vi "Q14070-Z060Abak.vi"() -> ()   [LabVIEW 2013]
uses:
  <vilib>/Utility/error.llb/whitespace.ctl
  <vilib>/Utility/file.llb/Read From Spreadsheet File (string).vi
  <vilib>/express/express arith-compare/Formula/XNode/ExpressFormulaBlockNode.xnode
  PCI8622_32.dll
  <vilib>/printing/EasyPrintingControls.llb/contents.ctl
  <vilib>/Utility/NIReport.llb/NI_ReportGenerationCore.lvlib
  <vilib>/printing/EasyPrintingControls.llb/report_type.ctl
  <vilib>/printing/EasyPrinting.llb/Easy Print VI Panel or Documentation (path).vi
  <vilib>/Utility/NIReport.llb/NI_report.lvclass
panel:
  in  "机械间隙值":dbl=3.5
  out "最大轴向力标准(N)":dbl=200.0 caption="L+Lmax(mm)" format="%#.3f"
  out "右平均轴向力(N)":dbl caption="L+Lmax(mm)" format="%#.3f"
  out "左平均轴向力(N)":dbl caption="最大位移偏离Lmax(mm)" format="%#.3f"
  out "员工ID":string
  out "急停":bool
  out "报警":dbl
  out "报警提示":string
  out "DeviceHandle":u32
  in  "设定轴向力调整次数":dbl=6.0
  out "出支线工步号":u32
  in  "最小间隙(mm)":dbl=0.001 format="%#.3f"
  in  "测头气缸右移":bool
  in  "测头气缸左移":bool
  in  "轴向力已做次数":dbl
  out "全行程间隙及轴向力合格":bool
  out "轴向力启动":bool
  out "间隙启动":bool
  in  "夹头松开":bool
  in  "夹头夹紧":bool
  out "找帽扭矩":dbl=8.0 caption="压力传感器" format="%#.2f"
  out "error out":errorcluster
  out "型号数量":i32
  out "error out 4":errorcluster
  in  "设定间隙调整次数":dbl=6.0
  out "读取产品ID":string
  out "下工位备料":bool
  out "下工位测试":bool
  out "下工位自动":bool
  out "下工位备料H":bool
  out "下工位测试H":bool
  out "下工位自动H":bool
  out "FGCS":string
  out "KSJJ":string
  out "Z060ARFID":string
  out "轴向力Y":dbl[](array[numeric])
  out "轴向力X":dbl[](array[numeric])
  out "间隙X数组":dbl[](array[numeric])
  out "间隙Y数组":dbl[](array[numeric])
  out "error out 3":errorcluster caption="错误输出"
  out "rfid工步号":u32
  out "芯片ID":string="201209190001"
  out "rfid完成":bool
  out "rfid触发":bool
  out "本序已做":bool
  in  "回零完成":bool
  in  "电动缸回零":bool
  in  "已调试次数":dbl
  in  "需调整角度(度)":dbl
  in  "转向器中心":dbl
  out "扭矩到达":bool
  out "黄灯":bool
  out "红灯":bool
  in  "基准位移":dbl caption="压力传感器" format="%#.3f"
  out "上序不合格":bool
  out "单点间隙合格":bool
  out "上序合格":bool
  out "测头机构电机":u32
  out "复位":bool
  in  "型号选择":u16(ring)=1 items=["J709", "J728", "J706"]
  in  "联线按钮":bool
  in  "工步号":u32
  in  "产品ID":string="201209190001"
  out "间隙位移(mm)":dbl caption="压力传感器" format="%#.3f"
  out "齿条推拉力(N)":dbl format="%#.2f"
  out "齿条扭矩(Nm)":dbl format="%#.2f"
  out "通讯状态":bool
  in  "员工ID":string
  out "员工姓名":string
  out "工步提示":string
  out "ADODB._Connection Out 2":refnum<k7>
  out "旋转齿条电机":u32
  out "电动缸电机":u32
  in  "停止":bool
  in  "参数加载":bool
  in  "选项卡控件":T1(tab)
  out "扭动曲线":cluster{"Y":dbl[], "Y":dbl[]}[](graph) caption="压球涨堵头1"
  out "中间位置间隙":dbl caption="间隙值L(mm)" format="%_2f"
  in  "中间间隙标准(mm)":dbl=0.07 format="%#.3f"
  in  "找帽OK":bool
  in  "全行程180°外间隙标准(mm)":dbl=0.1 format="%#.3f"
  out "右180°外全行程间隙":dbl caption="正向最大间隙L1(mm)" format="%_2f"
  out "左180°外全行程间隙":dbl caption="正向最大间隙L1(mm)" format="%_2f"
  out "右180°内全行程间隙":dbl caption="正向最大间隙L1(mm)" format="%_2f"
  out "左180°内全行程间隙":dbl caption="正向最大间隙L1(mm)" format="%_2f"
  in  "全行程180°内间隙标准(mm)":dbl=0.07 format="%_1f"
  out "左全行程间隙":dbl caption="正向最大间隙L1(mm)" format="%#.3f"
  out "右全行程间隙":dbl caption="正向最大间隙L1(mm)" format="%#.3f"
  out "总圈数最大值":dbl
  out "总圈数标准":dbl
  out "总行程最大值":dbl
  out "总行程标准(mm)":dbl
  out "平均轴向力MAX(N)":dbl=200.0 caption="L+Lmax(mm)" format="%#.3f"
  out "力波动标准(N)":dbl=60.0 caption="L+Lmax(mm)" format="%#.3f"
  out "轴向力标准(N)":dbl=100.0 caption="L+Lmax(mm)" format="%#.3f"
  out "右最大轴向力(N)":dbl caption="L+Lmax(mm)" format="%#_5f"
  out "左轴向力波动(N)":dbl caption="最大位移偏离Lmax(mm)" format="%#_4f"
  out "左最大轴向力(N)":dbl caption="最大位移偏离Lmax(mm)" format="%#_5f"
  out "行程跳动曲线":cluster{"Y":dbl[], "Y":dbl[]}[](graph) caption="压球涨堵头1"
  out "右轴向力波动(N)":dbl format="%#_4f"
  out "总行程(mm)":dbl format="%#_5f"
  out "总圈数":dbl format="%#.2f"
  in  "不合格品":bool
  in  "扭矩停止值":dbl=16.0
  in  "齿条右极限":dbl=-70.0 caption="压力传感器" format="%#.2f"
  in  "齿条左极限":dbl=-262.0 caption="压力传感器" format="%#.2f"
  in  "齿条移动速度":dbl=5.0 caption="压力传感器" format="%#.2f"
  in  "旋转伺服找帽转速":dbl=5.0 caption="压力传感器" format="%#.2f"
  in  "测量点扭矩":dbl=4.0 caption="压力传感器" format="%#.2f"
  in  "旋转伺服测量转速":dbl caption="压力传感器" format="%#.2f"
  in  "测头机构轴后退位":dbl=30.0 caption="压力传感器" format="%#.2f"
  in  "测头机构轴待检位":dbl caption="压力传感器" format="%#.2f"
  in  "测头机构轴检测位":dbl caption="压力传感器" format="%#.2f"
  in  "测头机构轴移动速度":dbl caption="压力传感器" format="%#.2f"
  out "点胶":bool
  in  "夹头松开":bool
  in  "夹头夹紧":bool
  in  "测头气缸右移":bool
  in  "测头气缸左移":bool
  in  "支线下降":bool
  in  "支线顶升":bool
  in  "出支线":bool
  in  "进支线":bool
  in  "主线下降":bool
  in  "主线顶升":bool
  in  "下阻挡器放行":bool
  in  "上阻挡器放行":bool
  out "夹头夹紧位":bool
  out "测头左位":bool
  out "测头右位":bool
  out "夹头松开":bool
  out "记号笔":bool
  in  "测头机构轴使能":bool
  in  "测头机构轴后退":bool
  in  "测头机构轴前进":bool
  in  "电动缸速度(mm/s)":dbl=10.0 format="%#.3f"
  out "电动缸位置(mm)":dbl=10000.0 format="%#.3f"
  in  "旋转伺服速度(°/s)":dbl=10.0 format="%#.3f"
  out "旋转伺服位置(°)":dbl=10000.0 format="%#.3f"
  in  "测头机构轴速度(mm/s)":dbl=10.0 format="%#.3f"
  out "测头机构轴位置(mm)":dbl=10000.0 format="%#.3f"
  in  "旋转齿条轴右转":bool
  in  "旋转齿条轴左转":bool
  in  "旋转齿条轴使能":bool
  in  "电动缸后退":bool
  in  "电动缸使能":bool
  in  "电动缸前进":bool
  in  "齿条扭矩比例偏移":dbl=1.0 format="%#.2f"
  in  "齿条扭矩零点偏移":dbl format="%#.2f"
  in  "齿条推拉力比例偏移":dbl=1.0 format="%#.2f"
  in  "齿条推拉力零点偏移":dbl format="%#.2f"
  in  "间隙位移比例偏移":dbl=1.0 format="%#.2f"
  in  "间隙位移零点偏移":dbl format="%#.2f"
  in  "传感器参数保存":bool
  in  "参数修改":bool
  in  "参数查询":bool
  in  "参数浏览表":string[][](table)
  # "芜湖机械转向器装配线"
  # "间隙及轴向力检测"
  # "Q14070机械转向器装配线"
  # "湖北唯思凌科装备制造有限公司 设计开发 (C)2015"
  # "≤"
  # "间隙测量判定值"
  # "间隙测量结果"
  # "≤"
  # "≤"
  # "≤"
  # "轴向力测量结果"
  # "轴向力测量标准"
  # "≤"
  # "≥"
  # "≤"
  # "≥"
  # "≤"
  # "≥"
  # "≤"
  # "不得大于20NM"
  # "传感器校验区"
  # "关于传感器校验：\n1、传感器校验需要由具备资质的单位或部门进行校验。\n2、具备权限的用户才能够修改传感器校验参数和试验参数。\n3、修改校验参数方法：先将比例偏移置为1，修改零点偏移，使零点值与校验的传感器一致；然后根据增幅调整比例偏移。"
  # "注意：\n具备权限的用户才能够修改传感器校验参数和试验参数！"
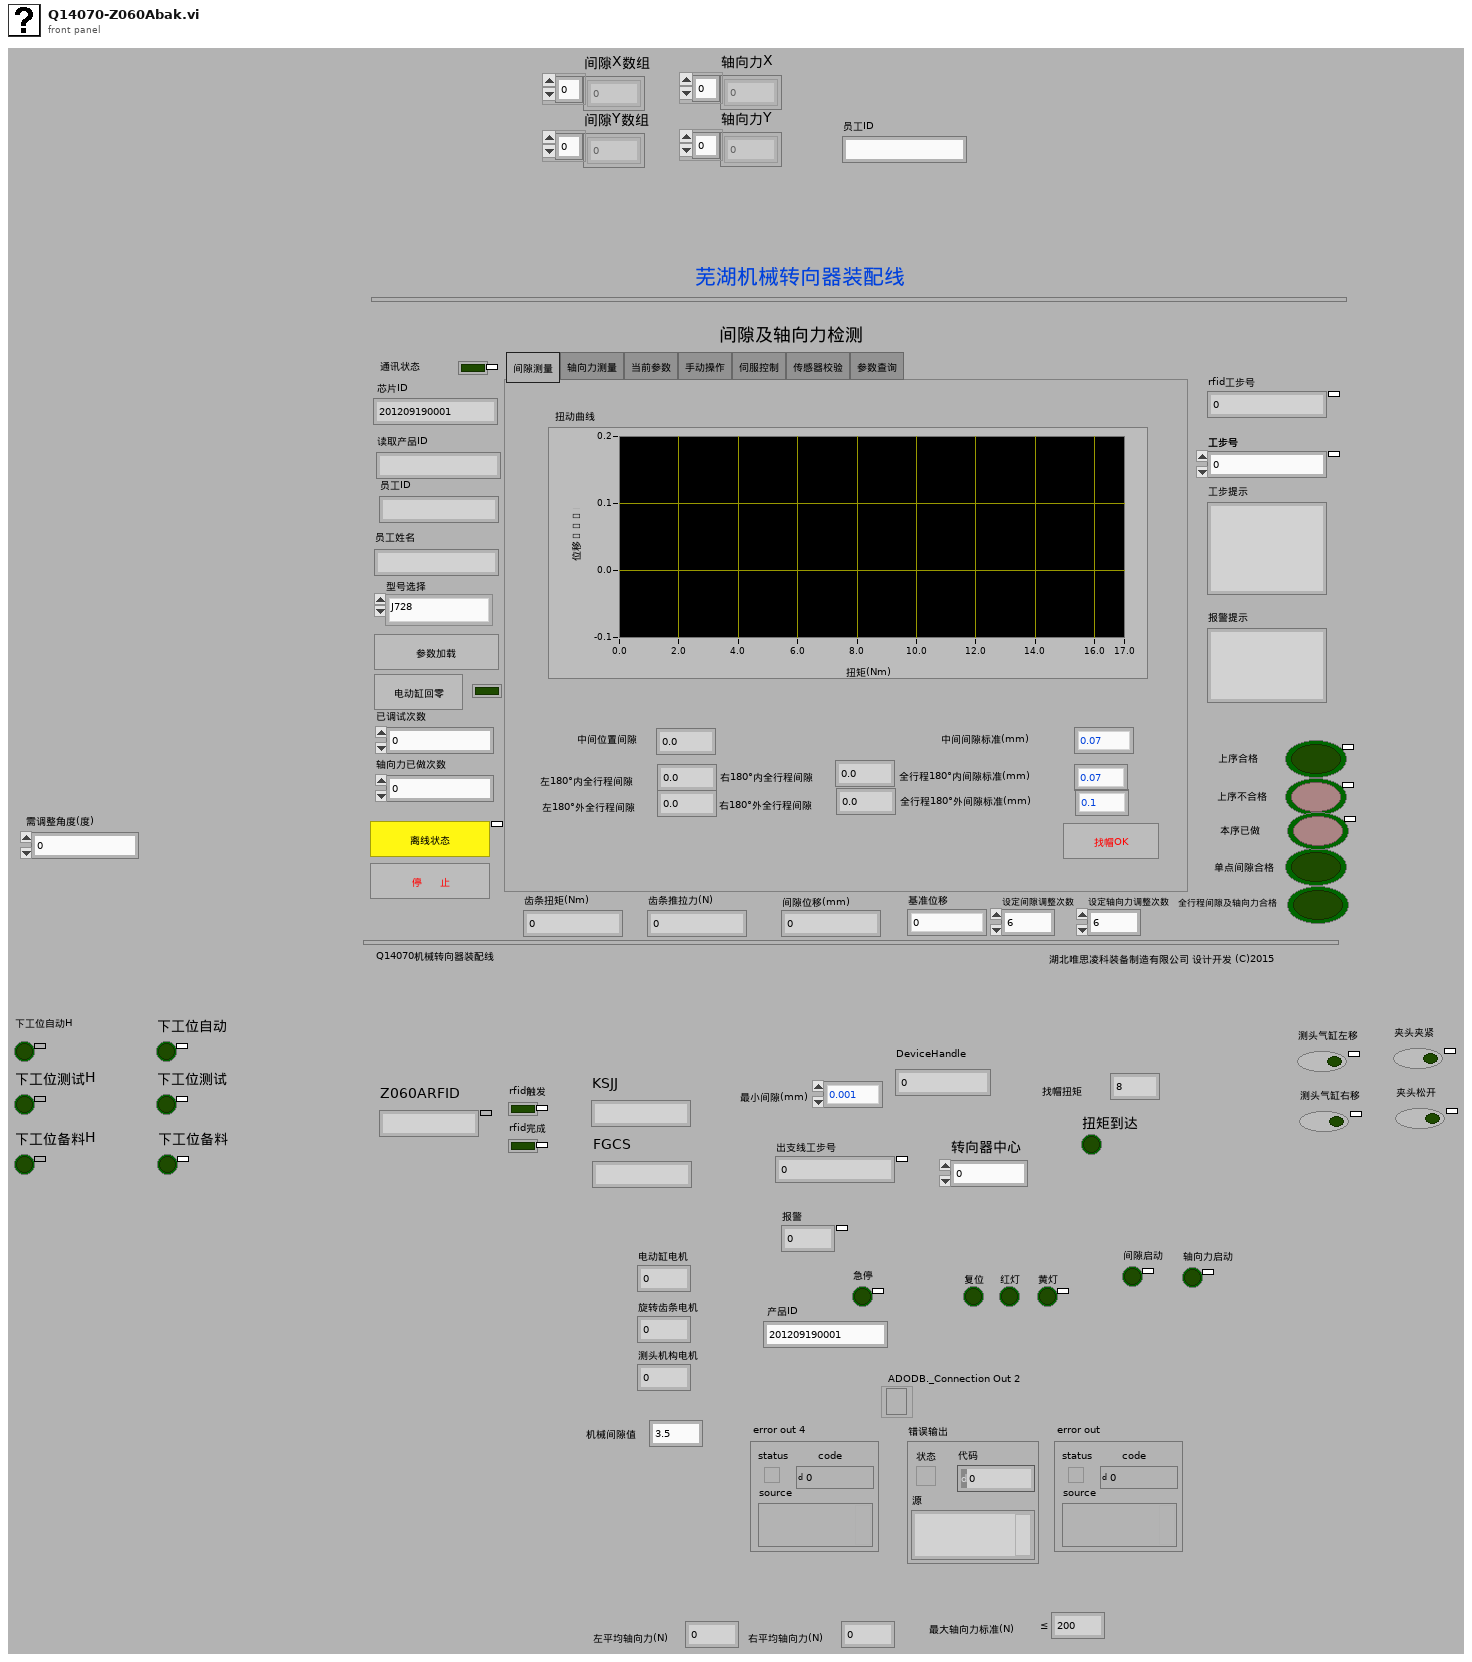
[diagram p1: front panel]
types:
  T1 = enum32{"间隙测量", "轴向力测量", "当前参数", "手动操作", "伺服控制", "传感器校验", "参数查询"}
  T2 = typedef "NI_ReportGenerationCore.lvlib/report_type.ctl" = u16
  T3 = typedef "NI_ReportGenerationCore.lvlib/contents.ctl" = u16
  T4 = typedef "imagedata.ctl" = cluster{"image type":i32, "image depth":i32, "image":u8[], "mask":u8[], "colors":u32[], "Rectangle":cluster{"left":i16, "top":i16, "right":i16, "bottom":i16}}
  T5 = enum8{"Enabled", "Disabled", "Disabled and Grayed Out"}
  T6 = typedef "whitespace.ctl" = u16
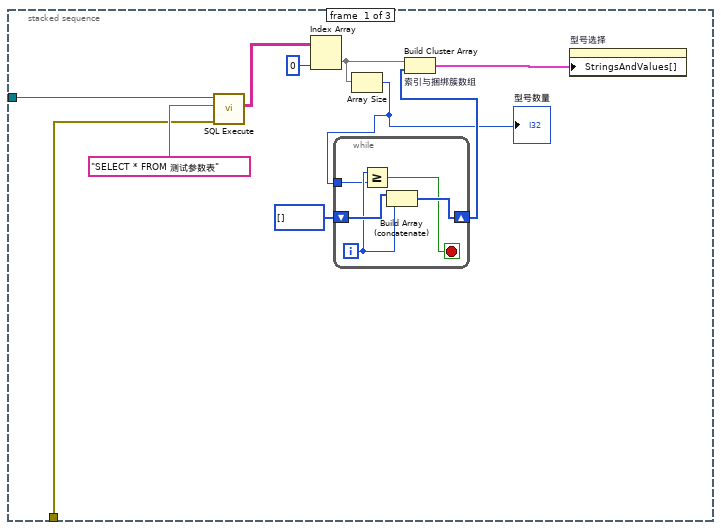
[diagram p4: hidden frame]
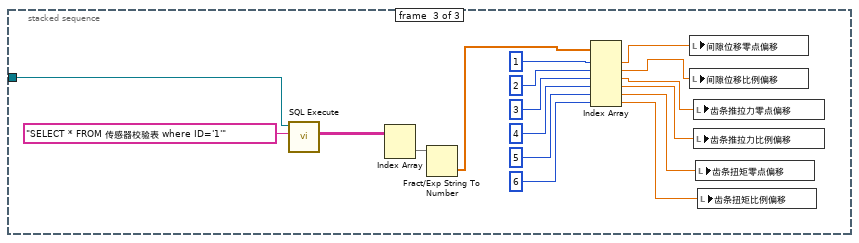
[diagram p5: hidden frame]
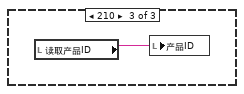
[diagram p7: hidden frame]
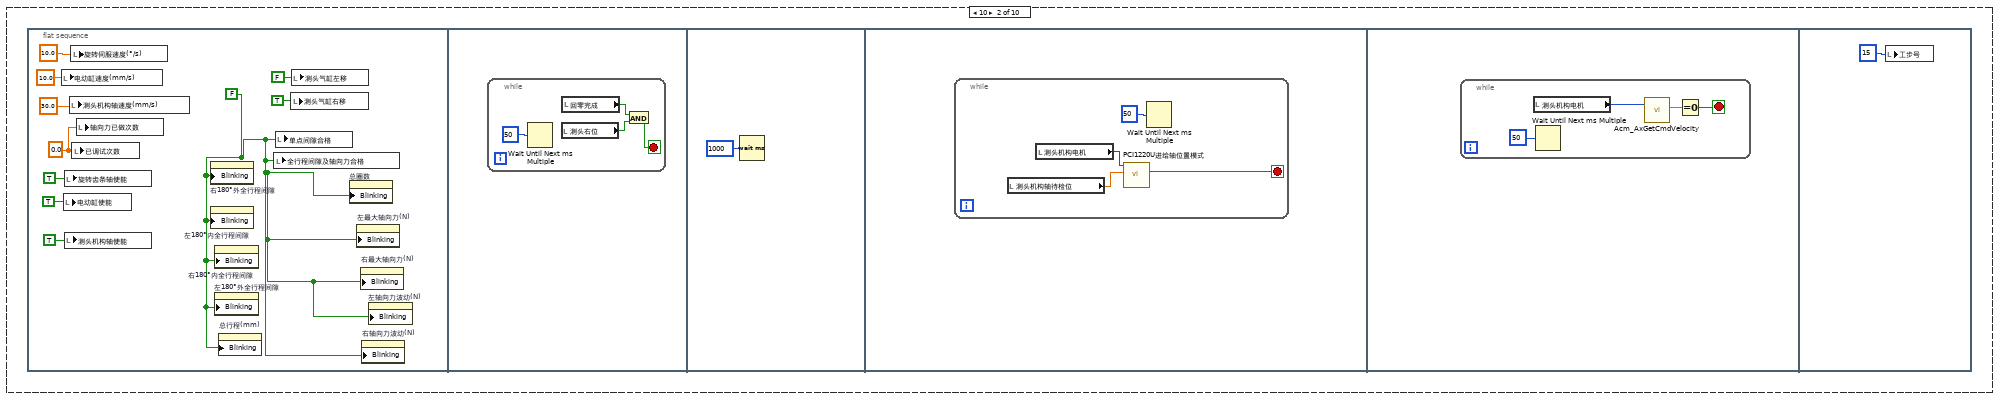
[diagram p8: hidden frame]
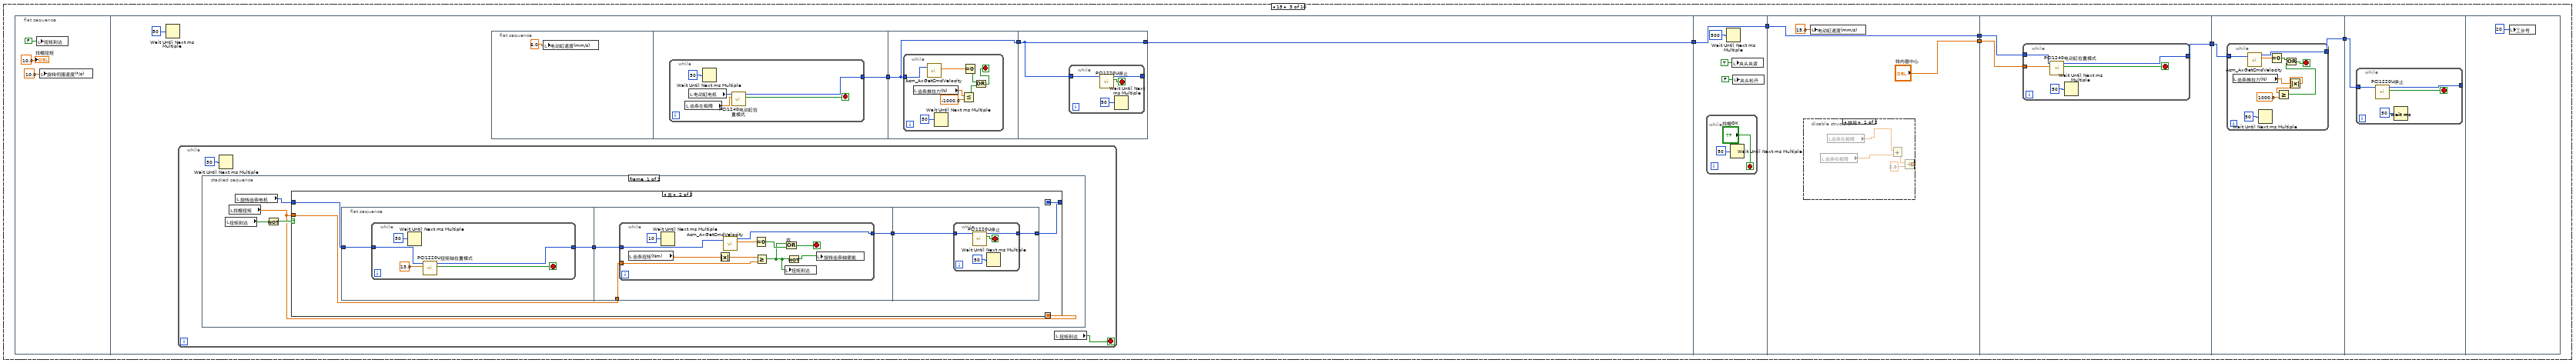
[diagram p9: hidden frame]
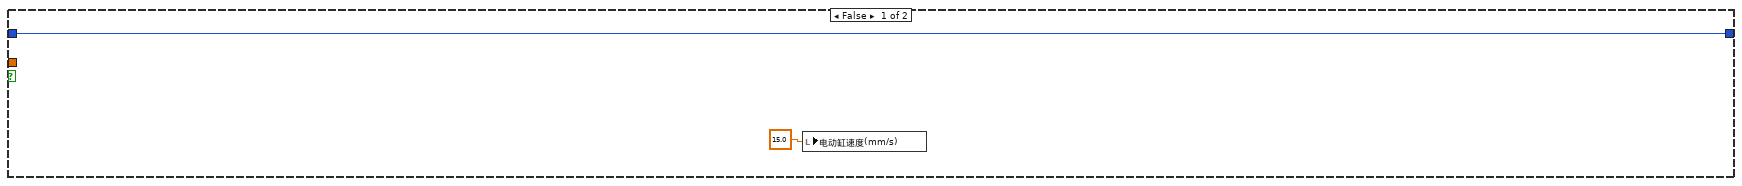
[diagram p10: hidden frame]
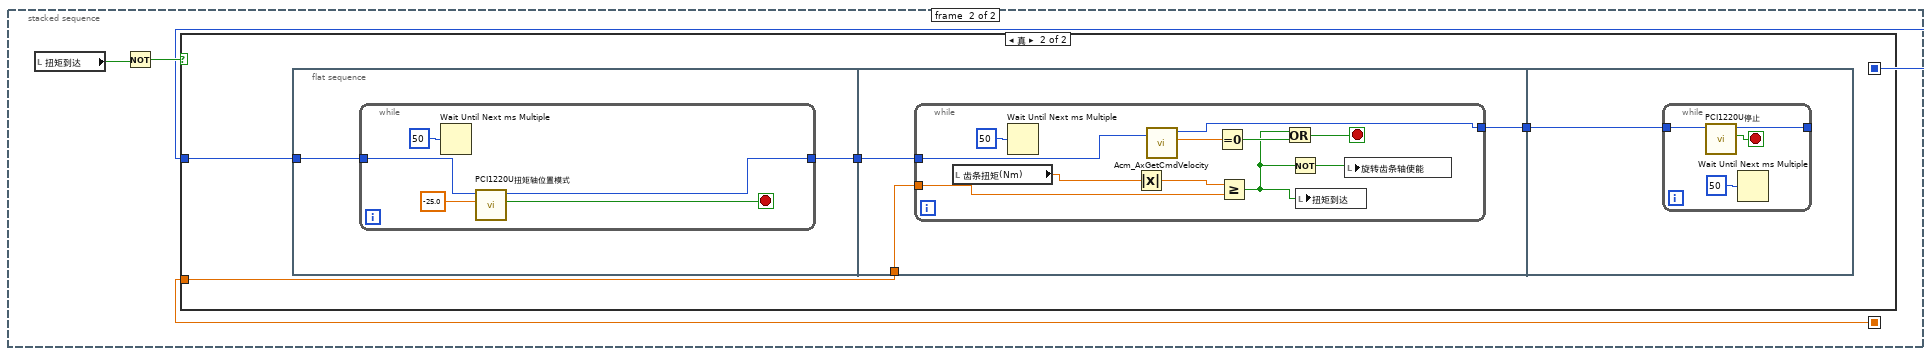
[diagram p11: hidden frame]
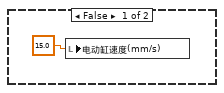
[diagram p12: hidden frame]
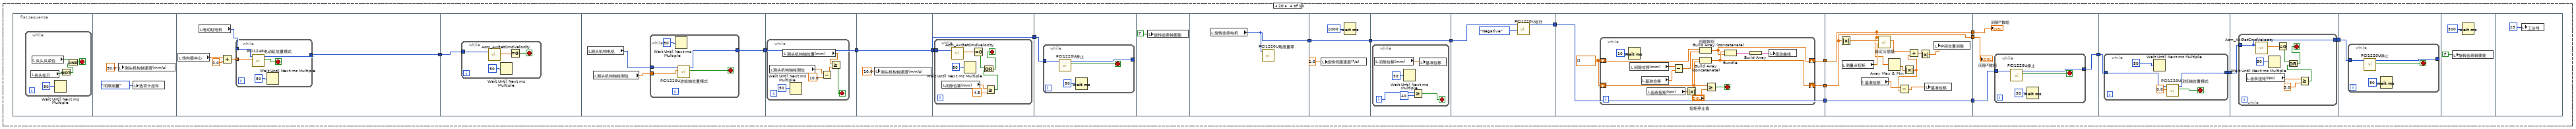
[diagram p14: hidden frame]
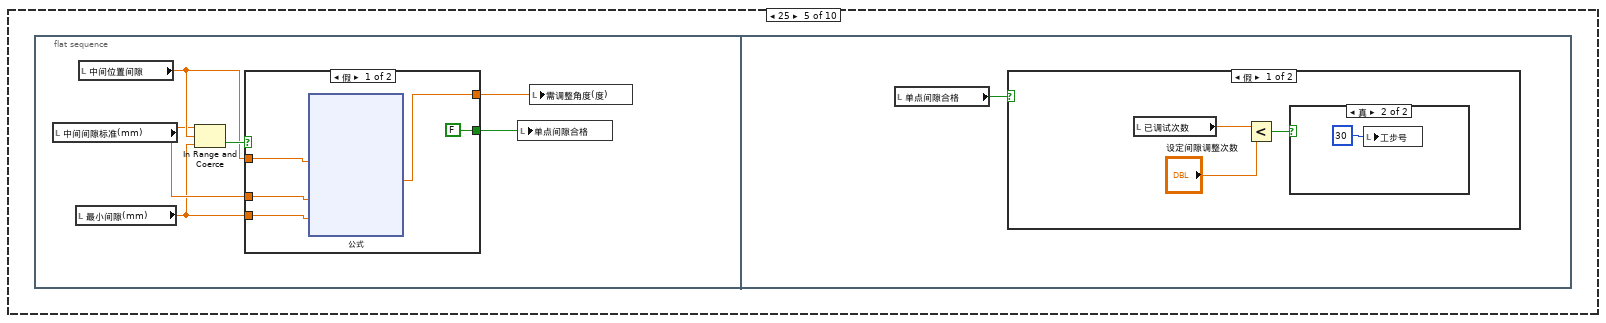
[diagram p15: hidden frame]
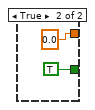
[diagram p16: hidden frame]
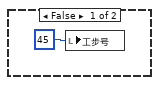
[diagram p17: hidden frame]
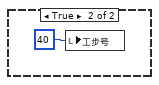
[diagram p18: hidden frame]
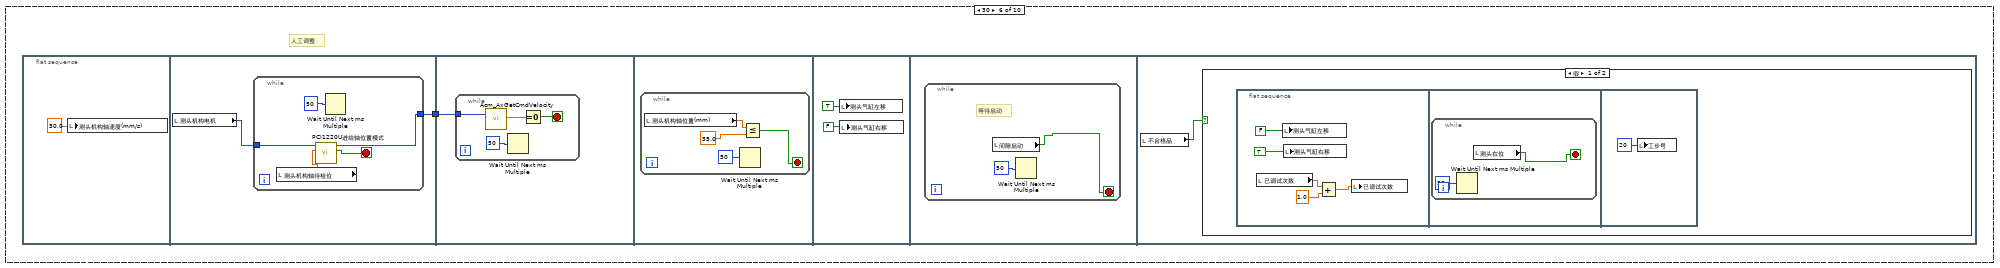
[diagram p19: hidden frame]
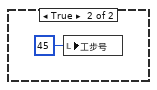
[diagram p20: hidden frame]
diagram:
  n1 = while {
    stop <- w7 stop-if-true
    n2 = local read "工步号"() -> (w5:u32)
    n3 = case shown="0, 默认" w5 {
      frame 0, Default {
        w8 = FALSE ("闪烁")
        n4 = property on="左最大轴向力(N)" class="DigNum (严格)"("Blinking"=w8) -> ()  [unwired: 2 in, 2 out]
        n5 = property on="右180°内全行程间隙" class="DigNum (严格)"("Blinking"=w8) -> ()  [unwired: 2 in, 2 out]
        n6 = property on="左180°内全行程间隙" class="DigNum (严格)"("Blinking"=w8) -> ()  [unwired: 2 in, 2 out]
        n7 = property on="右最大轴向力(N)" class="DigNum (严格)"("Blinking"=w8) -> ()  [unwired: 2 in, 2 out]
      }
      frame 10 {
        n8 = flat-sequence {
          frame #0 {
            w9 = FALSE ("单点间隙合格")
            w10 = 0.0 ("已调试次数")
            n9 = local write "电动缸速度(mm/s)"(10.0 ("电动缸速度(mm/s)")) -> ()
            n10 = local write "电动缸使能"(TRUE ("电动缸使能")) -> ()
            n11 = local write "旋转齿条轴使能"(TRUE ("旋转齿条轴使能")) -> ()
            n12 = local write "测头机构轴使能"(TRUE ("调整机构轴使能")) -> ()
            n13 = local write "测头机构轴速度(mm/s)"(30.0 ("调整机构轴速度(mm/s)")) -> ()
            n14 = local write "旋转伺服速度(°/s)"(10.0 ("旋转齿条轴速度(°/s)")) -> ()
            n15 = local write "已调试次数"(w10) -> ()
            n16 = local write "轴向力已做次数"(w10) -> ()
            n17 = property on="右180°外全行程间隙" class="DigNum (严格)"("Blinking"=w9) -> ()  [unwired: 2 in, 2 out]
            n18 = property on="左180°内全行程间隙" class="DigNum (严格)"("Blinking"=w9) -> ()  [unwired: 2 in, 2 out]
            n19 = property on="右180°内全行程间隙" class="DigNum (严格)"("Blinking"=w9) -> ()  [unwired: 2 in, 2 out]
            n20 = property on="左180°外全行程间隙" class="DigNum (严格)"("Blinking"=w9) -> ()  [unwired: 2 in, 2 out]
            n21 = property on="总行程(mm)" class="DigNum (严格)"("Blinking"=w9) -> ()  [unwired: 2 in, 2 out]
            n22 = local write "全行程间隙及轴向力合格"(w9) -> ()
            n23 = local write "单点间隙合格"(w9) -> ()
            n24 = local write "测头气缸右移"(TRUE ("测头气缸右移")) -> ()
            n25 = local write "测头气缸左移"(FALSE ("测头气缸左移")) -> ()
            n26 = property on="总圈数" class="DigNum (严格)"("Blinking"=w9) -> ()  [unwired: 2 in, 2 out]
            n27 = property on="左最大轴向力(N)" class="DigNum (严格)"("Blinking"=w9) -> ()  [unwired: 2 in, 2 out]
            n28 = property on="右最大轴向力(N)" class="DigNum (严格)"("Blinking"=w9) -> ()  [unwired: 2 in, 2 out]
            n29 = property on="右轴向力波动(N)" class="DigNum (严格)"("Blinking"=w9) -> ()  [unwired: 2 in, 2 out]
            n30 = property on="左轴向力波动(N)" class="DigNum (严格)"("Blinking"=w9) -> ()  [unwired: 2 in, 2 out]
          }
          frame #1 {
            n31 = while {
              stop <- w19 stop-if-true
              n32 = Wait Until Next ms Multiple(millisecond multiple=u32 50 ("毫秒倍数")) -> ()  [unwired: 1 out]
              n33 = local read "测头右位"() -> (w20:bool)
              n34 = local read "回零完成"() -> (w21:bool)
              n35 = And(x=w21, y=w20) -> (x .and. y?=w19:bool)
            }
          }
          frame #2 {
            n36 = Wait (ms)(milliseconds to wait=u32 1000 ("等待时间（毫秒）")) -> ()  [unwired: 1 out]
          }
          frame #3 {
            n37 = while {
              stop <- w27 stop-if-true
              n38 = local read "测头机构轴待检位"() -> (w24:dbl)
              n39 = local read "测头机构电机"() -> (w25:u32)
              n40 = call "PCI1220U进给轴位置模式.vi"("Distance"=w24, "AxisHandle IN"=w25) -> ("AbsSuccess"=w27:bool)  [unwired: 8 in, 1 out]
              n41 = Wait Until Next ms Multiple(millisecond multiple=u32 50 ("毫秒倍数")) -> ()  [unwired: 1 out]
            }
          }
          frame #4 {
            n42 = while {
              stop <- w30 stop-if-true
              n43 = local read "测头机构电机"() -> (w28:u32)
              n44 = Wait Until Next ms Multiple(millisecond multiple=u32 50 ("毫秒倍数")) -> ()  [unwired: 1 out]
              n45 = call <userlib>:"Acm_AxGetCmdVelocity.vi"("AxisHandle"=w28) -> ("Velocity"=w31:dbl)  [unwired: 1 in, 3 out]
              n46 = Equal To 0?(x=w31) -> (x = 0?=w30:bool)
            }
          }
          frame #5 {
            n47 = local write "工步号"(u32 15 ("工步号")) -> ()
          }
        }
      }
      frame 15 {
        n48 = flat-sequence {
          tunnel: [w43] -> w34
          tunnel: w34 -> [w145]
          tunnel: [w145] -> w35
          tunnel: [w150] -> w38
          tunnel: ["转向器中心"] -> w37
          tunnel: w35 -> [w150]
          tunnel: w38 -> [w159]
          tunnel: w37 -> [w158]
          tunnel: [w157] -> w36
          tunnel: w36 -> [w166]
          tunnel: [w165] -> w33
          tunnel: w33 -> [w177]
          frame #0 {
            n49 = local write "扭矩到达"(FALSE ("扭矩到达")) -> ()
            n50 = local write "旋转伺服速度(°/s)"(10.0 ("旋转齿条轴速度(°/s)")) -> ()
            "找帽扭矩" <- 10.0 ("找帽扭矩")
          }
          frame #1 {
            n51 = Wait Until Next ms Multiple(millisecond multiple=u32 50 ("毫秒倍数")) -> ()  [unwired: 1 out]
            n52 = while {
              stop <- w46 stop-if-true
              n53 = stacked-sequence {
                seq-local: [w48 _] -> [_ w89]
                seq-local: [w52 _] -> [_ w88]
                frame #0 {
                  n54 = local read "扭矩到达"() -> (w50:bool)
                  n55 = local read "找帽扭矩"() -> (w48:dbl)
                  n56 = local read "旋转齿条电机"() -> (w49:u32)
                  n57 = Not(x=w50) -> (.not. x?=w51:bool)
                  n58 = case shown="真" w51 {
                    tunnel: [w54 w55] -> w52
                    tunnel: w49 -> [w54 w59]
                    tunnel: w48 -> [_ w57]
                    frame False {
                      n59 = local write "电动缸速度(mm/s)"(15.0 ("电动缸速度(mm/s)")) -> ()
                    }
                    frame True {
                      n60 = flat-sequence {
                        tunnel: w59 -> [w61]
                        tunnel: [w60] -> w58
                        tunnel: w58 -> [w69]
                        tunnel: w57 -> [w68]
                        tunnel: [w67] -> w56
                        tunnel: w56 -> [w82]
                        tunnel: [w81] -> w55
                        frame #0 {
                          n61 = while {
                            tunnel: [w65] -> w60
                            tunnel: w61 -> [w62]
                            stop <- w64 stop-if-true
                            n62 = Wait Until Next ms Multiple(millisecond multiple=u32 50 ("毫秒倍数")) -> ()  [unwired: 1 out]
                            n63 = call "PCI1220U扭矩轴位置模式.vi"("Distance"=13.0, "AxisHandle IN"=w62) -> ("AbsSuccess"=w64:bool, "AxisHandle OUT"=w65:u32)  [unwired: 8 in]
                          }
                        }
                        frame #1 {
                          n64 = while {
                            tunnel: w69 -> [w79]
                            tunnel: w68 -> [w74]
                            tunnel: [w73] -> w67
                            stop <- w75 stop-if-true
                            n65 = local read "齿条扭矩(Nm)"() -> (w72:dbl)
                            n66 = Wait Until Next ms Multiple(millisecond multiple=u32 10 ("毫秒倍数")) -> ()  [unwired: 1 out]
                            n67 = Absolute Value(x=w72) -> (abs(x)=w77:dbl)
                            n68 = call <userlib>:"Acm_AxGetCmdVelocity.vi"("AxisHandle"=w79) -> ("Velocity"=w78:dbl, "AxisHandle"=w73:u32)  [unwired: 1 in, 2 out]
                            n69 = Equal To 0?(x=w78) -> (x = 0?=w76:bool)
                            n70 = Greater Or Equal?(x=w77, y=w74) -> (x >= y?=w71:bool)
                            n71 = Or "或"(x=w71, y=w76) -> (x .or. y?=w75:bool)
                            n72 = local write "扭矩到达"(w71) -> ()
                            n73 = Not(x=w71) -> (.not. x?=w70:bool)
                            n74 = local write "旋转齿条轴使能"(w70) -> ()
                          }
                        }
                        frame #2 {
                          n75 = while {
                            tunnel: w82 -> [w86]
                            tunnel: [w83] -> w81
                            stop <- w85 stop-if-true
                            n76 = call "PCI1220U停止.vi"("AxisHandle IN"=w86) -> ("完成"=w85:bool, "AxisHandle OUT"=w83:u32)  [unwired: 9 in]
                            n77 = Wait Until Next ms Multiple(millisecond multiple=u32 50 ("毫秒倍数")) -> ()  [unwired: 1 out]
                          }
                        }
                      }
                    }
                  }
                }
                frame #1 {
                  n78 = local read "扭矩到达"() -> (w87:bool)
                  n79 = Not(x=w87) -> (.not. x?=w90:bool)
                  n80 = case shown="真" w90 {
                    tunnel: w88 -> [_ w95]
                    tunnel: w89 -> [_ w93]
                    frame False {
                      n81 = local write "电动缸速度(mm/s)"(15.0 ("电动缸速度(mm/s)")) -> ()
                    }
                    frame True {
                      n82 = flat-sequence {
                        tunnel: w95 -> [w96]
                        tunnel: [w97] -> w94
                        tunnel: w94 -> [w105]
                        tunnel: w93 -> [w104]
                        tunnel: [w103] -> w92
                        tunnel: w92 -> [w117]
                        frame #0 {
                          n83 = while {
                            tunnel: [w101] -> w97
                            tunnel: w96 -> [w98]
                            stop <- w100 stop-if-true
                            n84 = Wait Until Next ms Multiple(millisecond multiple=u32 50 ("毫秒倍数")) -> ()  [unwired: 1 out]
                            n85 = call "PCI1220U扭矩轴位置模式.vi"("Distance"=-25.0, "AxisHandle IN"=w98) -> ("AbsSuccess"=w100:bool, "AxisHandle OUT"=w101:u32)  [unwired: 8 in]
                          }
                        }
                        frame #1 {
                          n86 = while {
                            tunnel: w105 -> [w115]
                            tunnel: [w110] -> w103
                            tunnel: w104 -> [w109]
                            stop <- w111 stop-if-true
                            n87 = local read "齿条扭矩(Nm)"() -> (w108:dbl)
                            n88 = Wait Until Next ms Multiple(millisecond multiple=u32 50 ("毫秒倍数")) -> ()  [unwired: 1 out]
                            n89 = Absolute Value(x=w108) -> (abs(x)=w113:dbl)
                            n90 = call <userlib>:"Acm_AxGetCmdVelocity.vi"("AxisHandle"=w115) -> ("Velocity"=w114:dbl, "AxisHandle"=w110:u32)  [unwired: 1 in, 2 out]
                            n91 = Equal To 0?(x=w114) -> (x = 0?=w112:bool)
                            n92 = Greater Or Equal?(x=w113, y=w109) -> (x >= y?=w106:bool)
                            n93 = Or(x=w106, y=w112) -> (x .or. y?=w111:bool)
                            n94 = Not(x=w106) -> (.not. x?=w107:bool)
                            n95 = local write "扭矩到达"(w106) -> ()
                            n96 = local write "旋转齿条轴使能"(w107) -> ()
                          }
                        }
                        frame #2 {
                          n97 = while {
                            tunnel: w117 -> [w121]
                            tunnel: [w118] -> _
                            stop <- w120 stop-if-true
                            n98 = call "PCI1220U停止.vi"("AxisHandle IN"=w121) -> ("完成"=w120:bool, "AxisHandle OUT"=w118:u32)  [unwired: 9 in]
                            n99 = Wait Until Next ms Multiple(millisecond multiple=u32 50 ("毫秒倍数")) -> ()  [unwired: 1 out]
                          }
                        }
                      }
                    }
                  }
                }
              }
              n100 = Wait Until Next ms Multiple(millisecond multiple=u32 50 ("毫秒倍数")) -> ()  [unwired: 1 out]
              n101 = local read "扭矩到达"() -> (w46:bool)
            }
            n102 = flat-sequence {
              tunnel: [w123] -> w45
              tunnel: w45 -> [w129]
              tunnel: [w129] -> w42
              tunnel: [w138] -> w43
              tunnel: w42 -> [w138]
              frame #0 {
                n103 = local write "电动缸速度(mm/s)"(6.0 ("电动缸速度(mm/s)")) -> ()
              }
              frame #1 {
                n104 = while {
                  tunnel: [w127] -> w123
                  stop <- w126 stop-if-true
                  n105 = local read "齿条左极限"() -> (w124:dbl)
                  n106 = local read "电动缸电机"() -> (w128:u32)
                  n107 = Wait Until Next ms Multiple(millisecond multiple=u32 50 ("毫秒倍数")) -> ()  [unwired: 1 out]
                  n108 = call "PCI1240电动缸位置模式 .vi"("Distance"=w124, "AxisHandle IN"=w128) -> ("AbsSuccess"=w126:bool, "AxisHandle OUT"=w127:u32)  [unwired: 8 in]
                }
              }
              frame #2 {
                n109 = while {
                  tunnel: w129 -> [w136]
                  stop <- w133 stop-if-true
                  n110 = local read "齿条推拉力(N)"() -> (w132:dbl)
                  n111 = call <userlib>:"Acm_AxGetCmdVelocity.vi"("AxisHandle"=w136) -> ("Velocity"=w137:dbl)  [unwired: 1 in, 3 out]
                  n112 = Wait Until Next ms Multiple(millisecond multiple=u32 50 ("毫秒倍数")) -> ()  [unwired: 1 out]
                  n113 = Less Or Equal?(x=w132, y=-1000.0) -> (x <= y?=w130:bool)
                  n114 = Equal To 0?(x=w137) -> (x = 0?=w134:bool)
                  n115 = Or(x=w134, y=w130) -> (x .or. y?=w133:bool)
                }
              }
              frame #3 {
                n116 = while {
                  tunnel: w138 -> [w142]
                  tunnel: [w139] -> _
                  stop <- w141 stop-if-true
                  n117 = call "PCI1220U停止.vi"("AxisHandle IN"=w142) -> ("完成"=w141:bool, "AxisHandle OUT"=w139:u32)  [unwired: 9 in]
                  n118 = Wait Until Next ms Multiple(millisecond multiple=u32 50 ("毫秒倍数")) -> ()  [unwired: 1 out]
                }
              }
            }
          }
          frame #2 {
            n119 = while {
              stop <- "找帽OK" stop-if-true
              n120 = Wait Until Next ms Multiple(millisecond multiple=u32 50 ("毫秒倍数")) -> ()  [unwired: 1 out]
            }
            n121 = Wait Until Next ms Multiple(millisecond multiple=u32 500 ("毫秒倍数")) -> ()  [unwired: 1 out]
            n122 = local write "夹头夹紧"(TRUE ("夹头夹紧")) -> ()
            n123 = local write "夹头松开"(FALSE ("夹头松开")) -> ()
          }
          frame #3 {
            n124 = disable-structure shown="禁用" {
              disable-tunnel: [w154 _] -> _
              frame Disabled {
                n125 = local read "齿条右极限"() -> (w152:dbl)
                n126 = local read "齿条左极限"() -> (w153:dbl)
                n127 = Add(x=w153, y=w152) -> (x+y=w156:dbl)
                n128 = Divide(x=w156, y=2.0) -> (x/y=w154:dbl)
              }
              frame Enabled {
              }
            }
            n129 = local write "电动缸速度(mm/s)"(15.0 ("电动缸轴移动速度")) -> ()
          }
          frame #4 {
            n130 = while {
              tunnel: w159 -> [w164]
              tunnel: w158 -> [w163]
              tunnel: [w160] -> w157
              stop <- w162 stop-if-true
              n131 = call "PCI1240电动缸位置模式 .vi"("Distance"=w163, "AxisHandle IN"=w164) -> ("AbsSuccess"=w162:bool, "AxisHandle OUT"=w160:u32)  [unwired: 8 in]
              n132 = Wait Until Next ms Multiple(millisecond multiple=u32 50 ("毫秒倍数")) -> ()  [unwired: 1 out]
            }
          }
          frame #5 {
            n133 = while {
              tunnel: w166 -> [w176]
              tunnel: [w167] -> w165
              stop <- w168 stop-if-true
              n134 = local read "齿条推拉力(N)"() -> (w173:dbl)
              n135 = call <userlib>:"Acm_AxGetCmdVelocity.vi"("AxisHandle"=w176) -> ("Velocity"=w175:dbl, "AxisHandle"=w167:u32)  [unwired: 1 in, 2 out]
              n136 = Wait Until Next ms Multiple(millisecond multiple=u32 50 ("毫秒倍数")) -> ()  [unwired: 1 out]
              n137 = Equal To 0?(x=w175) -> (x = 0?=w170:bool)
              n138 = Absolute Value(x=w173) -> (abs(x)=w172:dbl)
              n139 = Greater Or Equal?(x=w172, y=1000.0) -> (x >= y?=w169:bool)
              n140 = Or(x=w170, y=w169) -> (x .or. y?=w168:bool)
            }
          }
          frame #6 {
            n141 = while {
              tunnel: w177 -> [w181]
              tunnel: [w180] -> _
              stop <- w179 stop-if-true
              n142 = call "PCI1220U停止.vi"("AxisHandle IN"=w181) -> ("完成"=w179:bool, "AxisHandle OUT"=w180:u32)  [unwired: 9 in]
              n143 = Wait (ms)(milliseconds to wait=u32 50 ("毫秒倍数")) -> ()  [unwired: 1 out]
            }
          }
          frame #7 {
            n144 = local write "工步号"(u32 20 ("工步号")) -> ()
          }
        }
      }
      frame 20 {
        n145 = flat-sequence {
          tunnel: [w212] -> w193
          tunnel: w193 -> [w218]
          tunnel: [w224] -> w185
          tunnel: w185 -> [w231]
          tunnel: [w231] -> w184
          tunnel: w184 -> [w239]
          tunnel: [w239] -> w183
          tunnel: w183 -> [w240]
          tunnel: [w240] -> w192
          tunnel: w192 -> [w249]
          tunnel: [w255] -> w190
          tunnel: [w257] -> w191
          tunnel: w190 -> [w257]
          tunnel: [w259] -> w186
          tunnel: w191 -> [w259]
          tunnel: w186 -> [w266]
          tunnel: [w265] -> w197
          tunnel: [w270] -> w196
          tunnel: [w269] -> w195
          tunnel: w197 -> [w268]
          tunnel: [w268] -> w194
          tunnel: [w297] -> w200
          tunnel: [w294] -> w199
          tunnel: w196 -> [w294]
          tunnel: [w293] -> w198
          tunnel: w195 -> [w293]
          tunnel: w194 -> [w297]
          tunnel: w200 -> [w301]
          tunnel: [w300] -> w189
          tunnel: w199 -> [w298]
          tunnel: w198 -> [w299]
          tunnel: w189 -> [w307]
          tunnel: [w306] -> w188
          tunnel: w188 -> [w314]
          tunnel: [w313] -> w187
          tunnel: w187 -> [w323]
          frame #0 {
            n146 = while {
              stop <- w203 stop-if-true
              n147 = local read "夹头松开"() -> (w204:bool)
              n148 = local read "夹头夹紧位"() -> (w202:bool)
              n149 = Wait Until Next ms Multiple(millisecond multiple=u32 50 ("毫秒倍数")) -> ()  [unwired: 1 out]
              n150 = Not(x=w204) -> (.not. x?=w201:bool)
              n151 = And(x=w202, y=w201) -> (x .and. y?=w203:bool)
            }
          }
          frame #1 {
            n152 = local write "测头机构轴速度(mm/s)"(30.0 ("测头机构轴速度(mm/s)")) -> ()
            n153 = local write "选项卡控件"(T1."间隙测量" ("选项卡控件")) -> ()
          }
          frame #2 {
            n154 = local read "转向器中心"() -> (w210:dbl)
            n155 = local read "电动缸电机"() -> (w211:u32)
            n156 = Add(x=w210, y=0.0) -> (x+y=w209:dbl)
            n157 = while {
              tunnel: w211 -> [w217]
              tunnel: w209 -> [w216]
              tunnel: [w213] -> w212
              stop <- w215 stop-if-true
              n158 = call "PCI1240电动缸位置模式 .vi"("Distance"=w216, "AxisHandle IN"=w217) -> ("AbsSuccess"=w215:bool, "AxisHandle OUT"=w213:u32)  [unwired: 8 in]
              n159 = Wait Until Next ms Multiple(millisecond multiple=u32 50 ("毫秒倍数")) -> ()  [unwired: 1 out]
            }
          }
          frame #3 {
            n160 = while {
              tunnel: w218 -> [w222]
              stop <- w220 stop-if-true
              n161 = call <userlib>:"Acm_AxGetCmdVelocity.vi"("AxisHandle"=w222) -> ("Velocity"=w221:dbl)  [unwired: 1 in, 3 out]
              n162 = Wait Until Next ms Multiple(millisecond multiple=u32 50 ("毫秒倍数")) -> ()  [unwired: 1 out]
              n163 = Equal To 0?(x=w221) -> (x = 0?=w220:bool)
            }
          }
          frame #4 {
            n164 = local read "测头机构电机"() -> (w225:u32)
            n165 = local read "测头机构轴检测位"() -> (w223:dbl)
            n166 = while {
              tunnel: w225 -> [w228]
              tunnel: w223 -> [w227]
              tunnel: [w226] -> w224
              stop <- w230 stop-if-true
              n167 = Wait Until Next ms Multiple(millisecond multiple=u32 50 ("毫秒倍数")) -> ()  [unwired: 1 out]
              n168 = call "PCI1220U进给轴位置模式.vi"("Distance"=w227, "AxisHandle IN"=w228) -> ("AbsSuccess"=w230:bool, "AxisHandle OUT"=w226:u32)  [unwired: 8 in]
            }
          }
          frame #5 {
            n169 = while {
              stop <- w232 stop-if-true
              n170 = local read "测头机构轴检测位"() -> (w236:dbl)
              n171 = local read "测头机构轴位置(mm)"() -> (w235:dbl)
              n172 = Wait Until Next ms Multiple(millisecond multiple=u32 50 ("毫秒倍数")) -> ()  [unwired: 1 out]
              n173 = Subtract(x=w236, y=10.0) -> (x-y=w233:dbl)
              n174 = Greater Or Equal?(x=w235, y=w233) -> (x >= y?=w232:bool)
            }
          }
          frame #6 {
            n175 = local write "测头机构轴速度(mm/s)"(10.0 ("测头机构轴速度(mm/s)")) -> ()
          }
          frame #7 {
            n176 = while {
              tunnel: w240 -> [w248]
              stop <- w242 stop-if-true
              n177 = local read "间隙位移(mm)"() -> (w245:dbl)
              n178 = call <userlib>:"Acm_AxGetCmdVelocity.vi"("AxisHandle"=w248) -> ("Velocity"=w247:dbl)  [unwired: 1 in, 3 out]
              n179 = Wait Until Next ms Multiple(millisecond multiple=u32 50 ("毫秒倍数")) -> ()  [unwired: 1 out]
              n180 = Equal To 0?(x=w247) -> (x = 0?=w243:bool)
              n181 = Greater Or Equal?(x=w245, y=4.5) -> (x >= y?=w241:bool)
              n182 = Or(x=w243, y=w241) -> (x .or. y?=w242:bool)
            }
          }
          frame #8 {
            n183 = while {
              tunnel: w249 -> [w253]
              tunnel: [w252] -> _
              stop <- w251 stop-if-true
              n184 = call "PCI1220U停止.vi"("AxisHandle IN"=w253) -> ("完成"=w251:bool, "AxisHandle OUT"=w252:u32)  [unwired: 9 in]
              n185 = Wait (ms)(milliseconds to wait=u32 50 ("毫秒倍数")) -> ()  [unwired: 1 out]
            }
          }
          frame #9 {
            n186 = local write "旋转齿条轴使能"(TRUE ("旋转齿条轴使能")) -> ()
          }
          frame #10 {
            n187 = local read "旋转齿条电机"() -> (w255:u32)
            n188 = call "PCI1220U角度置零.vi"("AxisHandle IN"=w255) -> ()  [unwired: 10 in, 1 out]
          }
          frame #11 {
            n189 = local write "旋转伺服速度(°/s)"(1.0 ("旋转齿条轴速度(°/s)")) -> ()
            n190 = Wait (ms)(milliseconds to wait=u32 1000 ("毫秒倍数")) -> ()  [unwired: 1 out]
          }
          frame #12 {
            n191 = while {
              i -> [w263]
              stop <- w260 stop-if-true
              n192 = local read "间隙位移(mm)"() -> (w264:dbl)
              n193 = Wait Until Next ms Multiple(millisecond multiple=u32 50 ("毫秒倍数")) -> ()  [unwired: 1 out]
              n194 = Greater Or Equal?(x=w263, y=40) -> (x >= y?=w260:bool)
              n195 = local write "基准位移"(w264) -> ()
            }
          }
          frame #13 {
            n196 = call "PCI1220U运行.vi"("方向"=enum32{"Negative", "Positive"}."Negative" ("Direction"), "AxisHandle IN"=w266) -> ("AxisHandle OUT"=w265:u32)  [unwired: 9 in]
          }
          frame #14 {
            w271 = dbl[] []
            n197 = while {
              shift-right: [w282] -> w270
              shift-left: w271 -> [w284]
              shift-right: [w281] -> w269
              shift-left: w271 -> [w283]
              stop <- w274 stop-if-true
              n198 = Wait (ms)(milliseconds to wait=u32 10 ("毫秒倍数")) -> ()  [unwired: 1 out]
              n199 = local read "间隙位移(mm)"() -> (w277:dbl)
              n200 = local read "基准位移"() -> (w275:dbl)
              n201 = local read "齿条扭矩(Nm)"() -> (w278:dbl)
              n202 = Subtract(x=w277, y=w275) -> (x-y=w276:dbl)
              n203 = Absolute Value(x=w278) -> (abs(x)=w273:dbl)
              n204 = Build Array (concatenate) "创建数组"(w283, w276) -> (w281:dbl[])
              n205 = Build Array (concatenate) ("创建数组")(w284, w273) -> (w282:dbl[])
              n206 = Greater Or Equal?(x=w273, y="扭矩停止值") -> (x >= y?=w274:bool)
              n207 = Bundle ("捆绑")(w282, w281) -> (w279:cluster{dbl[], dbl[]})  [unwired: 1 in]
              n208 = Build Array ("创建数组")(w279) -> (w280:cluster{dbl[], dbl[]}[])
              n209 = local write "扭动曲线"(w280) -> ()
            }
          }
          frame #15 {
            n210 = Absolute Value(x=w294) -> (abs(x)=w295:dbl[])
            n211 = local read "测量点扭矩"() -> (w296:dbl)
            n212 = local read "基准位移"() -> (w290:dbl)
            n213 = call "自定义插值.vi"("压力"=w296, "扭矩数组"=w295, "位移数组"=w293) -> ("扭矩值"=w291:dbl)  [unwired: 8 in]
            n214 = Array Max & Min(array=w293) -> (min value=w292:dbl)  [unwired: 3 out]
            n215 = Absolute Value(x=w292) -> (abs(x)=w289:dbl)
            n216 = Subtract(x=w290, y=w289) -> (x-y=w288:dbl)
            n217 = Add(x=w291, y=w289) -> (x+y=w287:dbl)
            n218 = Absolute Value(x=w287) -> (abs(x)=w286:dbl)
            n219 = local write "基准位移"(w288) -> ()
            n220 = local write "中间位置间隙"(w286) -> ()
          }
          frame #16 {
            n221 = while {
              tunnel: w301 -> [w305]
              tunnel: [w304] -> w300
              stop <- w303 stop-if-true
              n222 = call "PCI1220U停止.vi"("AxisHandle IN"=w305) -> ("完成"=w303:bool, "AxisHandle OUT"=w304:u32)  [unwired: 9 in]
              n223 = Wait (ms)(milliseconds to wait=u32 50 ("毫秒倍数")) -> ()  [unwired: 1 out]
            }
            "间隙Y数组" <- w299
            "间隙X数组" <- w298
          }
          frame #17 {
            n224 = while {
              tunnel: [w312] -> w306
              tunnel: w307 -> [w309]
              stop <- w311 stop-if-true
              n225 = Wait Until Next ms Multiple(millisecond multiple=u32 50 ("毫秒倍数")) -> ()  [unwired: 1 out]
              n226 = call "PCI1220U扭矩轴位置模式.vi"("Distance"=0.0, "AxisHandle IN"=w309) -> ("AbsSuccess"=w311:bool, "AxisHandle OUT"=w312:u32)  [unwired: 8 in]
            }
          }
          frame #18 {
            n227 = while {
              tunnel: w314 -> [w316]
              tunnel: [w316] -> w313
              stop <- w319 stop-if-true
              n228 = local read "齿条扭矩(Nm)"() -> (w315:dbl)
              n229 = call <userlib>:"Acm_AxGetCmdVelocity.vi"("AxisHandle"=w316) -> ("Velocity"=w322:dbl)  [unwired: 1 in, 3 out]
              n230 = Wait Until Next ms Multiple(millisecond multiple=u32 50 ("毫秒倍数")) -> ()  [unwired: 1 out]
              n231 = Equal To 0?(x=w322) -> (x = 0?=w320:bool)
              n232 = Greater Or Equal?(x=w315, y=3.0) -> (x >= y?=w317:bool)
              n233 = Or(x=w320, y=w317) -> (x .or. y?=w319:bool)
            }
          }
          frame #19 {
            n234 = while {
              tunnel: w323 -> [w327]
              tunnel: [w326] -> _
              stop <- w325 stop-if-true
              n235 = call "PCI1220U停止.vi"("AxisHandle IN"=w327) -> ("完成"=w325:bool, "AxisHandle OUT"=w326:u32)  [unwired: 9 in]
              n236 = Wait (ms)(milliseconds to wait=u32 50 ("毫秒倍数")) -> ()  [unwired: 1 out]
            }
          }
          frame #20 {
            n237 = local write "旋转齿条轴使能"(FALSE ("旋转齿条轴使能")) -> ()
            n238 = Wait (ms)(milliseconds to wait=u32 500 ("毫秒倍数")) -> ()  [unwired: 1 out]
          }
          frame #21 {
            n239 = local write "工步号"(u32 25 ("工步号")) -> ()
          }
        }
      }
      frame 25 {
        n240 = flat-sequence {
          frame #0 {
            n241 = local read "中间间隙标准(mm)"() -> (w332:dbl)
            n242 = local read "最小间隙(mm)"() -> (w331:dbl)
            n243 = local read "中间位置间隙"() -> (w333:dbl)
            n244 = In Range and Coerce(upper limit=w332, x=w333, lower limit=w331) -> (In Range?=w336:bool)  [unwired: 1 out]
            n245 = case shown="假" w336 {
              tunnel: [FALSE ("本序合格") TRUE ("本序合格")] -> w335
              tunnel: [w341 0.0 ("需调整角度(度)")] -> w334
              tunnel: w333 -> [w339 _]
              tunnel: w332 -> [w338 _]
              tunnel: w331 -> [w337 _]
              frame False {
                n246 = xnode "公式"("X"=w339, "Xmax"=w338, "Xmin"=w337) -> ("结果"=w341:dbl)  [unwired: 1 in, 1 out]
              }
              frame True {
              }
            }
            n247 = local write "单点间隙合格"(w335) -> ()
            n248 = local write "需调整角度(度)"(w334) -> ()
          }
          frame #1 {
            n249 = local read "单点间隙合格"() -> (w356:bool)
            n250 = case shown="假" w356 {
              frame False {
                n251 = local read "已调试次数"() -> (w359:dbl)
                n252 = Less?(x=w359, y="设定间隙调整次数") -> (x < y?=w358:bool)
                n253 = case shown="真" w358 {
                  frame False {
                    n254 = local write "工步号"(u32 45 ("变更工步号")) -> ()
                  }
                  frame True {
                    n255 = local write "工步号"(u32 30 ("变更工步号")) -> ()
                  }
                }
              }
              frame True {
                n256 = local write "工步号"(u32 40 ("变更工步号")) -> ()
              }
            }
          }
        }
      }
      frame 30 {
        # "人工调整"
        n257 = flat-sequence {
          tunnel: [w365] -> w363
          tunnel: w363 -> [w372]
          frame #0 {
            n258 = local write "测头机构轴速度(mm/s)"(30.0 ("测头机构轴速度(mm/s)")) -> ()
          }
          frame #1 {
            n259 = local read "测头机构电机"() -> (w366:u32)
            n260 = while {
              tunnel: w366 -> [w369]
              tunnel: [w368] -> w365
              stop <- w371 stop-if-true
              n261 = local read "测头机构轴待检位"() -> (w367:dbl)
              n262 = call "PCI1220U进给轴位置模式.vi"("Distance"=w367, "AxisHandle IN"=w369) -> ("AbsSuccess"=w371:bool, "AxisHandle OUT"=w368:u32)  [unwired: 8 in]
              n263 = Wait Until Next ms Multiple(millisecond multiple=u32 50 ("毫秒倍数")) -> ()  [unwired: 1 out]
            }
          }
          frame #2 {
            n264 = while {
              tunnel: w372 -> [w376]
              stop <- w374 stop-if-true
              n265 = call <userlib>:"Acm_AxGetCmdVelocity.vi"("AxisHandle"=w376) -> ("Velocity"=w375:dbl)  [unwired: 1 in, 3 out]
              n266 = Wait Until Next ms Multiple(millisecond multiple=u32 50 ("毫秒倍数")) -> ()  [unwired: 1 out]
              n267 = Equal To 0?(x=w375) -> (x = 0?=w374:bool)
            }
          }
          frame #3 {
            n268 = while {
              stop <- w378 stop-if-true
              n269 = local read "测头机构轴位置(mm)"() -> (w380:dbl)
              n270 = Wait Until Next ms Multiple(millisecond multiple=u32 50 ("毫秒倍数")) -> ()  [unwired: 1 out]
              n271 = Less Or Equal?(x=w380, y=35.0) -> (x <= y?=w378:bool)
            }
          }
          frame #4 {
            n272 = local write "测头气缸左移"(TRUE ("测头气缸左移")) -> ()
            n273 = local write "测头气缸右移"(FALSE ("测头气缸右移")) -> ()
          }
          frame #5 {
            n274 = while {
              stop <- w383 stop-if-true
              # "等待启动"
              n275 = local read "间隙启动"() -> (w383:bool)
              n276 = Wait Until Next ms Multiple(millisecond multiple=u32 50 ("毫秒倍数")) -> ()  [unwired: 1 out]
            }
          }
          frame #6 {
            n277 = local read "不合格品"() -> (w385:bool)
            n278 = case shown="假" w385 {
              frame False {
                n279 = flat-sequence {
                  frame #0 {
                    n280 = local read "已调试次数"() -> (w388:dbl)
                    n281 = local write "测头气缸左移"(FALSE ("测头气缸左移")) -> ()
                    n282 = local write "测头气缸右移"(TRUE ("测头气缸左移")) -> ()
                    n283 = Add(x=w388, y=1.0 ("已调试次数")) -> (x+y=w390:dbl)
                    n284 = local write "已调试次数"(w390) -> ()
                  }
                  frame #1 {
                    n285 = while {
                      stop <- w391 stop-if-true
                      n286 = Wait Until Next ms Multiple(millisecond multiple=u32 50 ("毫秒倍数")) -> ()  [unwired: 1 out]
                      n287 = local read "测头右位"() -> (w391:bool)
                    }
                  }
                  frame #2 {
                    n288 = local write "工步号"(u32 20 ("工步号")) -> ()
                  }
                }
              }
              frame True {
                n289 = local write "工步号"(u32 45 ("工步号")) -> ()
              }
            }
          }
        }
      }
      frame 40 {
        n290 = flat-sequence {
          tunnel: [w557] -> w553
          tunnel: w553 -> [w559]
          tunnel: [w558] -> w467
          tunnel: w467 -> [w565]
          tunnel: [w565] -> w466
          tunnel: w466 -> [w575]
          tunnel: [w575] -> w469
          tunnel: w469 -> [w576]
          tunnel: [w577] -> w468
          tunnel: w468 -> [w583]
          tunnel: [w583] -> w544
          tunnel: w544 -> [w592]
          tunnel: [w592] -> w543
          tunnel: w543 -> [w599]
          tunnel: [w599] -> w551
          tunnel: w551 -> [w601]
          tunnel: [w602] -> w465
          tunnel: [w600] -> w463
          tunnel: w465 -> [w611]
          tunnel: [w611] -> w464
          tunnel: w463 -> [w612]
          tunnel: [w612] -> w462
          tunnel: [w610] -> w459
          tunnel: [w609] -> w456
          tunnel: [w608] -> w453
          tunnel: w464 -> [w651]
          tunnel: [w651] -> w471
          tunnel: w462 -> [w650]
          tunnel: [w650] -> w470
          tunnel: [w648] -> w460
          tunnel: w459 -> [w648]
          tunnel: [w647] -> w457
          tunnel: w456 -> [w647]
          tunnel: [w646] -> w454
          tunnel: w453 -> [w646]
          tunnel: w471 -> [w657]
          tunnel: [w657] -> w473
          tunnel: w470 -> [w656]
          tunnel: [w655] -> w472
          tunnel: [w654] -> w461
          tunnel: w460 -> [w654]
          tunnel: [w653] -> w458
          tunnel: w457 -> [w653]
          tunnel: [w652] -> w455
          tunnel: w454 -> [w652]
          tunnel: [w671] -> w549
          tunnel: [w670] -> w548
          tunnel: [w669] -> w547
          tunnel: w473 -> [w668]
          tunnel: [w668] -> w546
          tunnel: [w667] -> w545
          tunnel: w472 -> [w666]
          tunnel: w461 -> [w665]
          tunnel: w458 -> [w664]
          tunnel: w455 -> [w663]
          tunnel: w549 -> [w711]
          tunnel: [w711] -> w523
          tunnel: w548 -> [w718]
          tunnel: [w718] -> w521
          tunnel: w547 -> [w714]
          tunnel: [w714] -> w519
          tunnel: w546 -> [w717]
          tunnel: [w717] -> w517
          tunnel: [w713] -> w515
          tunnel: w545 -> [w713]
          tunnel: [w715] -> w513
          tunnel: [w705] -> w511
          tunnel: [w712] -> w509
          tunnel: [w706] -> w507
          tunnel: [w710] -> w505
          tunnel: [w709] -> w503
          tunnel: [w707] -> w502
          tunnel: [w708] -> w501
          tunnel: [w704] -> w478
          tunnel: w523 -> [w741]
          tunnel: [w741] -> w522
          tunnel: w521 -> [w740]
          tunnel: [w740] -> w520
          tunnel: w519 -> [w739]
          tunnel: [w739] -> w518
          tunnel: w517 -> [w738]
          tunnel: [w738] -> w516
          tunnel: w515 -> [w737]
          tunnel: [w737] -> w514
          tunnel: w513 -> [w736]
          tunnel: [w736] -> w512
          tunnel: w511 -> [w735]
          tunnel: [w735] -> w510
          tunnel: w509 -> [w734]
          tunnel: [w734] -> w508
          tunnel: w507 -> [w733]
          tunnel: [w733] -> w506
          tunnel: w505 -> [w732]
          tunnel: [w732] -> w504
          tunnel: w503 -> [w727]
          tunnel: w502 -> [w729]
          tunnel: w501 -> [w728]
          tunnel: w478 -> [w726]
          tunnel: [w724] -> w412
          tunnel: [w723] -> w395
          tunnel: w522 -> [w760]
          tunnel: [w760] -> w448
          tunnel: w520 -> [w759]
          tunnel: [w759] -> w447
          tunnel: w518 -> [w758]
          tunnel: [w758] -> w446
          tunnel: w516 -> [w757]
          tunnel: [w757] -> w445
          tunnel: [w756] -> w444
          tunnel: w514 -> [w756]
          tunnel: [w755] -> w443
          tunnel: w512 -> [w755]
          tunnel: w510 -> [w751]
          tunnel: w508 -> [w754]
          tunnel: w506 -> [w752]
          tunnel: w504 -> [w753]
          tunnel: [w753] -> w442
          tunnel: [w745] -> w441
          tunnel: [w744] -> w440
          tunnel: w412 -> [w743]
          tunnel: [w743] -> w411
          tunnel: [w742] -> w396
          tunnel: w395 -> [w742]
          tunnel: w448 -> [w775]
          tunnel: w447 -> [w774]
          tunnel: w446 -> [w773]
          tunnel: w445 -> [w768]
          tunnel: w444 -> [w772]
          tunnel: w443 -> [w779]
          tunnel: [w779] -> w439
          tunnel: w442 -> [w778]
          tunnel: [w778] -> w437
          tunnel: w441 -> [w777]
          tunnel: [w777] -> w435
          tunnel: w440 -> [w776]
          tunnel: [w776] -> w433
          tunnel: [w771] -> w430
          tunnel: [w770] -> w427
          tunnel: [w769] -> w424
          tunnel: [w768] -> w421
          tunnel: [w767] -> w417
          tunnel: w411 -> [w766]
          tunnel: [w766] -> w410
          tunnel: [w765] -> w397
          tunnel: w396 -> [w765]
          tunnel: w439 -> [w823]
          tunnel: [w823] -> w438
          tunnel: w437 -> [w822]
          tunnel: [w822] -> w436
          tunnel: w435 -> [w821]
          tunnel: [w821] -> w434
          tunnel: w433 -> [w820]
          tunnel: [w820] -> w432
          tunnel: [w818] -> w431
          tunnel: w430 -> [w818]
          tunnel: [w817] -> w428
          tunnel: w427 -> [w817]
          tunnel: [w816] -> w425
          tunnel: w424 -> [w816]
          tunnel: [w815] -> w422
          tunnel: w421 -> [w815]
          tunnel: [w814] -> w418
          tunnel: w417 -> [w814]
          tunnel: w410 -> [w813]
          tunnel: [w813] -> w409
          tunnel: [w812] -> w398
          tunnel: w397 -> [w812]
          tunnel: w438 -> [w834]
          tunnel: [w834] -> w452
          tunnel: w436 -> [w833]
          tunnel: [w833] -> w451
          tunnel: w434 -> [w832]
          tunnel: [w832] -> w450
          tunnel: w432 -> [w831]
          tunnel: [w831] -> w449
          tunnel: w431 -> [w828]
          tunnel: [w830] -> w429
          tunnel: w428 -> [w830]
          tunnel: [w829] -> w426
          tunnel: w425 -> [w829]
          tunnel: [w828] -> w423
          tunnel: w422 -> [w827]
          tunnel: [w827] -> w420
          tunnel: [w826] -> w419
          tunnel: w418 -> [w826]
          tunnel: w409 -> [w825]
          tunnel: [w825] -> w408
          tunnel: [w824] -> w399
          tunnel: w398 -> [w824]
          tunnel: [w853] -> w542
          tunnel: [w852] -> w541
          tunnel: [w851] -> w539
          tunnel: w452 -> [w849]
          tunnel: [w850] -> w537
          tunnel: [w849] -> w535
          tunnel: w451 -> [w848]
          tunnel: [w848] -> w526
          tunnel: w450 -> [w847]
          tunnel: w449 -> [w846]
          tunnel: [w847] -> w491
          tunnel: [w846] -> w490
          tunnel: w429 -> [w845]
          tunnel: w426 -> [w844]
          tunnel: w423 -> [w843]
          tunnel: w420 -> [w842]
          tunnel: w419 -> [w841]
          tunnel: w408 -> [w840]
          tunnel: [w840] -> w407
          tunnel: [w839] -> w400
          tunnel: w399 -> [w839]
          tunnel: w542 -> [w891]
          tunnel: w541 -> [w899]
          tunnel: [w899] -> w540
          tunnel: w539 -> [w896]
          tunnel: [w896] -> w538
          tunnel: w537 -> [w898]
          tunnel: [w898] -> w536
          tunnel: w535 -> [w897]
          tunnel: [w897] -> w534
          tunnel: [w893] -> w528
          tunnel: [w892] -> w527
          tunnel: w526 -> [w890]
          tunnel: [w891] -> w525
          tunnel: [w890] -> w524
          tunnel: w491 -> [w889]
          tunnel: w490 -> [w888]
          tunnel: [w889] -> w486
          tunnel: [w888] -> w483
          tunnel: w407 -> [w887]
          tunnel: [w887] -> w406
          tunnel: [w886] -> w401
          tunnel: w400 -> [w886]
          tunnel: w540 -> [w935]
          tunnel: [w946] -> w552
          tunnel: w538 -> [w946]
          tunnel: w536 -> [w945]
          tunnel: w534 -> [w944]
          tunnel: [w942] -> w533
          tunnel: w528 -> [w941]
          tunnel: w527 -> [w940]
          tunnel: w525 -> [w923]
          tunnel: w524 -> [w922]
          tunnel: [w931] -> w500
          tunnel: [w930] -> w489
          tunnel: [w929] -> w487
          tunnel: w486 -> [w929]
          tunnel: [w928] -> w484
          tunnel: w483 -> [w928]
          tunnel: [w927] -> w481
          tunnel: [w926] -> w479
          tunnel: [w909] -> w476
          tunnel: [w910] -> w474
          tunnel: [w908] -> w416
          tunnel: [w907] -> w414
          tunnel: w406 -> [w905]
          tunnel: [w905] -> w405
          tunnel: [w904] -> w402
          tunnel: w401 -> [w904]
          tunnel: w552 -> [w971]
          tunnel: [w971] -> w499
          tunnel: [w967] -> w497
          tunnel: w533 -> [w969]
          tunnel: [w966] -> w495
          tunnel: w500 -> [w965]
          tunnel: [w953] -> w493
          tunnel: [w963] -> w492
          tunnel: w489 -> [w962]
          tunnel: [w957] -> w488
          tunnel: w487 -> [w957]
          tunnel: [w956] -> w485
          tunnel: w484 -> [w956]
          tunnel: [w955] -> w482
          tunnel: w481 -> [w955]
          tunnel: [w954] -> w480
          tunnel: w479 -> [w954]
          tunnel: [w952] -> w477
          tunnel: w476 -> [w952]
          tunnel: [w951] -> w475
          tunnel: w474 -> [w951]
          tunnel: w416 -> [w950]
          tunnel: [w950] -> w415
          tunnel: w414 -> [w949]
          tunnel: [w949] -> w413
          tunnel: w405 -> [w948]
          tunnel: [w948] -> w404
          tunnel: [w947] -> w403
          tunnel: w402 -> [w947]
          tunnel: w499 -> [w988]
          tunnel: [w988] -> w498
          tunnel: w497 -> [w987]
          tunnel: [w987] -> w496
          tunnel: w495 -> [w986]
          tunnel: [w986] -> w494
          tunnel: w493 -> [w982]
          tunnel: w492 -> [w978]
          tunnel: w488 -> [w981]
          tunnel: w485 -> [w980]
          tunnel: w482 -> [w984]
          tunnel: w480 -> [w983]
          tunnel: w477 -> [w977]
          tunnel: w475 -> [w976]
          tunnel: w415 -> [w975]
          tunnel: w413 -> [w974]
          tunnel: w404 -> [w973]
          tunnel: w403 -> [w972]
          tunnel: w498 -> [w992]
          tunnel: [w991] -> w550
          tunnel: w496 -> [w990]
          tunnel: [w989] -> w529
          tunnel: w494 -> [w989]
          tunnel: w550 -> [w999]
          tunnel: [w999] -> w532
          tunnel: [w998] -> w530
          tunnel: w529 -> [w998]
          tunnel: w532 -> [w1006]
          tunnel: [w1005] -> w531
          tunnel: w530 -> [w1004]
          tunnel: w531 -> [w1012]
          frame #0 {
            n291 = local write "电动缸速度(mm/s)"(15.0 ("电动缸速度(mm/s)")) -> ()
            n292 = local write "已调试次数"(0.0 ("已调试次数")) -> ()
            n293 = local write "选项卡控件"(T1."轴向力测量" ("选项卡控件")) -> ()
            n294 = local read "电动缸电机"() -> (w557:u32)
          }
          frame #1 {
            n295 = while {
              tunnel: w559 -> [w564]
              tunnel: [w563] -> w558
              stop <- w562 stop-if-true
              n296 = local read "齿条左极限"() -> (w560:dbl)
              n297 = Wait (ms)(milliseconds to wait=u32 50 ("毫秒倍数")) -> ()  [unwired: 1 out]
              n298 = call "PCI1240电动缸位置模式 .vi"("Distance"=w560, "AxisHandle IN"=w564) -> ("AbsSuccess"=w562:bool, "AxisHandle OUT"=w563:u32)  [unwired: 8 in]
            }
          }
          frame #2 {
            n299 = while {
              tunnel: w565 -> [w573]
              stop <- w566 stop-if-true
              n300 = local read "齿条推拉力(N)"() -> (w570:dbl)
              n301 = call <userlib>:"Acm_AxGetCmdVelocity.vi"("AxisHandle"=w573) -> ("Velocity"=w572:dbl)  [unwired: 1 in, 3 out]
              n302 = Wait Until Next ms Multiple(millisecond multiple=u32 50 ("毫秒倍数")) -> ()  [unwired: 1 out]
              n303 = Equal To 0?(x=w572) -> (x = 0?=w568:bool)
              n304 = Less Or Equal?(x=w570, y=-300.0) -> (x <= y?=w567:bool)
              n305 = Or ("或")(x=w568, y=w567) -> (x .or. y?=w566:bool)
            }
          }
          frame #3 {
            n306 = local write "电动缸速度(mm/s)"(1.0 ("电动缸速度(mm/s)")) -> ()
          }
          frame #4 {
            n307 = while {
              tunnel: [w581] -> w577
              tunnel: w576 -> [w580]
              stop <- w582 stop-if-true
              n308 = Wait (ms)(milliseconds to wait=u32 50 ("毫秒倍数")) -> ()  [unwired: 1 out]
              n309 = call "PCI1240电动缸位置模式 .vi"("Distance"=118.0, "AxisHandle IN"=w580) -> ("AbsSuccess"=w582:bool, "AxisHandle OUT"=w581:u32)  [unwired: 8 in]
            }
          }
          frame #5 {
            n310 = while {
              tunnel: w583 -> [w591]
              stop <- w584 stop-if-true
              n311 = local read "齿条推拉力(N)"() -> (w588:dbl)
              n312 = call <userlib>:"Acm_AxGetCmdVelocity.vi"("AxisHandle"=w591) -> ("Velocity"=w590:dbl)  [unwired: 1 in, 3 out]
              n313 = Wait Until Next ms Multiple(millisecond multiple=u32 50 ("毫秒倍数")) -> ()  [unwired: 1 out]
              n314 = Equal To 0?(x=w590) -> (x = 0?=w586:bool)
              n315 = Less Or Equal?(x=w588, y=-300.0) -> (x <= y?=w585:bool)
              n316 = Or ("或")(x=w586, y=w585) -> (x .or. y?=w584:bool)
            }
          }
          frame #6 {
            n317 = while {
              tunnel: w592 -> [w596]
              tunnel: [w595] -> _
              stop <- w594 stop-if-true
              n318 = call "PCI1220U停止.vi"("AxisHandle IN"=w596) -> ("完成"=w594:bool, "AxisHandle OUT"=w595:u32)  [unwired: 9 in]
              n319 = Wait (ms)(milliseconds to wait=u32 50 ("毫秒倍数")) -> ()  [unwired: 1 out]
            }
          }
          frame #7 {
            n320 = Wait Until Next ms Multiple(millisecond multiple=u32 50 ("毫秒倍数")) -> ()  [unwired: 1 out]
            n321 = local write "电动缸速度(mm/s)"(15.0 ("电动缸速度(mm/s)")) -> ()
          }
          frame #8 {
            n322 = while {
              tunnel: w601 -> [w607]
              tunnel: [w604] -> w600
              stop <- w605 stop-if-true
              n323 = local read "齿条右极限"() -> (w603:dbl)
              n324 = Wait Until Next ms Multiple(millisecond multiple=u32 50 ("毫秒倍数")) -> ()  [unwired: 1 out]
              n325 = call "PCI1240电动缸位置模式 .vi"("Distance"=w603, "AxisHandle IN"=w607) -> ("AbsSuccess"=w605:bool, "AxisHandle OUT"=w604:u32)  [unwired: 8 in]
            }
            n326 = local read "转向器中心"() -> (w602:dbl)
          }
          frame #9 {
            w613 = dbl[] []
            n327 = while {
              shift-right: [w634] -> w609
              shift-left: w613 -> [w644]
              shift-right: [w642] -> w610
              shift-left: w613 -> [w643]
              tunnel: w612 -> [w639]
              tunnel: [w639] -> _
              tunnel: w611 -> [w637]
              shift-right: [w633] -> w608
              shift-left: w613 -> [w635]
              stop <- w627 stop-if-true
              n328 = local read "中间位置间隙"() -> (w624:dbl)
              n329 = local read "基准位移"() -> (w640:dbl)
              n330 = local read "间隙位移(mm)"() -> (w623:dbl)
              n331 = call <userlib>:"Acm_AxGetCmdVelocity.vi"("AxisHandle"=w639) -> ("Velocity"=w632:dbl)  [unwired: 1 in, 3 out]
              n332 = Wait (ms)(milliseconds to wait=u32 50 ("毫秒倍数")) -> ()  [unwired: 1 out]
              n333 = local read "齿条推拉力(N)"() -> (w630:dbl)
              n334 = call "PCI1240电动缸读取位置.vi"("AxisHandle IN"=w639) -> ("位置"=w638:dbl)  [unwired: 9 in, 1 out]
              n335 = Subtract(x=w623, y=w640) -> (x-y=w626:dbl)
              n336 = Subtract(x=w638, y=w637) -> (x-y=w617:dbl)
              n337 = Add(x=w626, y=w624) -> (x+y=w625:dbl)
              n338 = Multiply(x=w617, y=1.12) -> (x*y=w615:dbl)
              n339 = Build Array (concatenate) ("创建数组")(w643, w625) -> (w642:dbl[])
              n340 = Build Array (concatenate) ("创建数组")(w644, w615) -> (w634:dbl[])
              n341 = Build Array (concatenate) ("创建数组")(w635, w630) -> (w633:dbl[])
              n342 = Greater Or Equal?(x=w630, y=300.0) -> (x >= y?=w628:bool)
              n343 = Less Or Equal?(x=w623, y=0.0) -> (x <= y?=w622:bool)
              n344 = Greater Or Equal?(x=w623, y=4.0) -> (x >= y?=w621:bool)
              n345 = Equal To 0?(x=w632) -> (x = 0?=w629:bool)
              n346 = Or(x=w621, y=w622) -> (x .or. y?=w620:bool)
              n347 = Bundle ("捆绑")(w634, w642) -> (w614:cluster{dbl[], dbl[]})  [unwired: 1 in]
              n348 = Or(x=w629, y=w628) -> (x .or. y?=w627:bool)
              n349 = Bundle ("捆绑")(w634, w633) -> (w636:cluster{dbl[], dbl[]})  [unwired: 1 in]
              n350 = property on="间隙位移(mm)" class="DigNum (严格)"("Blinking"=w620) -> ()  [unwired: 2 in, 2 out]
              n351 = Build Array ("创建数组")(w614, w636) -> (w641:cluster{dbl[], dbl[]}[])
              n352 = local write "行程跳动曲线"(w641) -> ()
            }
          }
          frame #10 {
            n353 = local write "电动缸速度(mm/s)"(1.0 ("电动缸速度(mm/s)")) -> ()
          }
          frame #11 {
            n354 = while {
              tunnel: w656 -> [w660]
              tunnel: [w659] -> w655
              stop <- w662 stop-if-true
              n355 = Wait Until Next ms Multiple(millisecond multiple=u32 50 ("毫秒倍数")) -> ()  [unwired: 1 out]
              n356 = call "PCI1240电动缸位置模式 .vi"("Distance"=-30.0, "AxisHandle IN"=w660) -> ("AbsSuccess"=w662:bool, "AxisHandle OUT"=w659:u32)  [unwired: 8 in]
            }
          }
          frame #12 {
            n357 = while {
              shift-right: [w692] -> w670
              shift-left: w664 -> [w702]
              shift-right: [w700] -> w671
              shift-left: w665 -> [w701]
              tunnel: w666 -> [w697]
              tunnel: [w697] -> w669
              tunnel: w668 -> [w695]
              shift-right: [w691] -> w667
              shift-left: w663 -> [w693]
              stop <- w685 stop-if-true
              n358 = local read "中间位置间隙"() -> (w682:dbl)
              n359 = local read "基准位移"() -> (w698:dbl)
              n360 = local read "间隙位移(mm)"() -> (w681:dbl)
              n361 = call <userlib>:"Acm_AxGetCmdVelocity.vi"("AxisHandle"=w697) -> ("Velocity"=w690:dbl)  [unwired: 1 in, 3 out]
              n362 = Wait (ms)(milliseconds to wait=u32 50 ("毫秒倍数")) -> ()  [unwired: 1 out]
              n363 = local read "齿条推拉力(N)"() -> (w688:dbl)
              n364 = call "PCI1240电动缸读取位置.vi"("AxisHandle IN"=w697) -> ("位置"=w696:dbl)  [unwired: 9 in, 1 out]
              n365 = Subtract(x=w681, y=w698) -> (x-y=w684:dbl)
              n366 = Subtract(x=w696, y=w695) -> (x-y=w675:dbl)
              n367 = Add(x=w684, y=w682) -> (x+y=w683:dbl)
              n368 = Multiply(x=w675, y=1.12) -> (x*y=w673:dbl)
              n369 = Build Array (concatenate) ("创建数组")(w701, w683) -> (w700:dbl[])
              n370 = Build Array (concatenate) ("创建数组")(w702, w673) -> (w692:dbl[])
              n371 = Build Array (concatenate) ("创建数组")(w693, w688) -> (w691:dbl[])
              n372 = Greater Or Equal?(x=w688, y=300.0) -> (x >= y?=w686:bool)
              n373 = Less Or Equal?(x=w681, y=0.0) -> (x <= y?=w680:bool)
              n374 = Greater Or Equal?(x=w681, y=4.0) -> (x >= y?=w679:bool)
              n375 = Equal To 0?(x=w690) -> (x = 0?=w687:bool)
              n376 = Or(x=w679, y=w680) -> (x .or. y?=w678:bool)
              n377 = Bundle ("捆绑")(w692, w700) -> (w672:cluster{dbl[], dbl[]})  [unwired: 1 in]
              n378 = Or(x=w687, y=w686) -> (x .or. y?=w685:bool)
              n379 = Bundle ("捆绑")(w692, w691) -> (w694:cluster{dbl[], dbl[]})  [unwired: 1 in]
              n380 = property on="间隙位移(mm)" class="DigNum (严格)"("Blinking"=w678) -> ()  [unwired: 2 in, 2 out]
              n381 = Build Array ("创建数组")(w672, w694) -> (w699:cluster{dbl[], dbl[]}[])
              n382 = local write "行程跳动曲线"(w699) -> ()
            }
          }
          frame #13 {
            n383 = Wait Until Next ms Multiple(millisecond multiple=u32 500 ("毫秒倍数")) -> ()  [unwired: 1 out]
            n384 = while {
              tunnel: w714 -> [w722]
              tunnel: [w721] -> _
              stop <- w720 stop-if-true
              n385 = call "PCI1220U停止.vi"("AxisHandle IN"=w722) -> ("完成"=w720:bool, "AxisHandle OUT"=w721:u32)  [unwired: 9 in]
              n386 = Wait (ms)(milliseconds to wait=u32 50 ("毫秒倍数")) -> ()  [unwired: 1 out]
            }
            n387 = Array Size(array=w713) -> (size(s)=w715:i32)
            n388 = call "间隙计算.vi"("扭矩数组"=w711) -> ("峰值间隙1"=w707:dbl, "峰值间隙2"=w708:dbl)  [unwired: 6 in, 3 out]
            n389 = call "功能计算.vi"("扭矩数组"=w713) -> ("扭差"=w706:dbl, "平均扭矩"=w712:dbl, "峰值扭矩"=w705:dbl)  [unwired: 7 in, 1 out]
            n390 = Array Size(array=w711) -> (size(s)=w710:i32)
            n391 = local read "全行程180°外间隙标准(mm)"() -> (w704:dbl)
            n392 = local read "全行程180°内间隙标准(mm)"() -> (w709:dbl)
            n393 = local write "左180°内全行程间隙"(w707) -> ()
            n394 = local write "左180°外全行程间隙"(w708) -> ()
            n395 = local write "左最大轴向力(N)"(w705) -> ()
            n396 = local write "左平均轴向力(N)"(w712) -> ()
            n397 = local write "左轴向力波动(N)"(w706) -> ()
          }
          frame #14 {
            n398 = Less?(x=w728, y=w726) -> (x < y?=w730:bool)
            n399 = Less?(x=w729, y=w727) -> (x < y?=w731:bool)
            n400 = Not(x=w730) -> (.not. x?=w723:bool)
            n401 = local write "电动缸速度(mm/s)"(15.0 ("电动缸速度(mm/s)")) -> ()
            n402 = Not(x=w731) -> (.not. x?=w724:bool)
            n403 = property on="左180°外全行程间隙" class="DigNum (严格)"("Blinking"=w723) -> ()  [unwired: 2 in, 2 out]
            n404 = property on="左180°内全行程间隙" class="DigNum (严格)"("Blinking"=w724) -> ()  [unwired: 2 in, 2 out]
          }
          frame #15 {
            n405 = local read "最大轴向力标准(N)"() -> (w749:dbl)
            n406 = while {
              tunnel: w758 -> [w764]
              tunnel: w757 -> [_]
              stop <- w763 stop-if-true
              n407 = local read "齿条左极限"() -> (w761:dbl)
              n408 = Wait Until Next ms Multiple(millisecond multiple=u32 50 ("毫秒倍数")) -> ()  [unwired: 1 out]
              n409 = call "PCI1240电动缸位置模式 .vi"("Distance"=w761, "AxisHandle IN"=w764) -> ("AbsSuccess"=w763:bool)  [unwired: 8 in, 1 out]
            }
            n410 = local read "轴向力标准(N)"() -> (w748:dbl)
            n411 = local read "平均轴向力MAX(N)"() -> (w747:dbl)
            n412 = local read "力波动标准(N)"() -> (w746:dbl)
            n413 = call "判断.vi"("y 3"=w746, "y2-2"=w747, "y2-1"=w748, "y"=w749, "x 3"=w752, "x 2"=w754, "x"=w751) -> ("非x? 3"=w744:bool, "非x? 2"=w750:bool, "非x?"=w745:bool)  [unwired: 2 in]
            n414 = property on="左最大轴向力(N)" class="DigNum (严格)"("Blinking"=w745) -> ()  [unwired: 2 in, 2 out]
            n415 = property on="左轴向力波动(N)" class="DigNum (严格)"("Blinking"=w744) -> ()  [unwired: 2 in, 2 out]
            n416 = property on="左平均轴向力(N)" class="DigNum (严格)"("Blinking"=w750) -> ()  [unwired: 2 in, 2 out]
          }
          frame #16 {
            n417 = while {
              shift-right: [w781] -> w769
              shift-left: w774 -> [w810]
              shift-right: [w808] -> w770
              shift-left: w775 -> [w809]
              tunnel: w773 -> [w805]
              tunnel: [w805] -> w771
              tunnel: w768 -> [w803]
              shift-right: [w800] -> w767
              shift-left: w772 -> [w801]
              stop <- w795 stop-if-true
              n418 = local read "间隙位移(mm)"() -> (w787:dbl)
              n419 = call <userlib>:"Acm_AxGetCmdVelocity.vi"("AxisHandle"=w805) -> ("Velocity"=w793:dbl)  [unwired: 1 in, 3 out]
              n420 = local read "基准位移"() -> (w806:dbl)
              n421 = Wait (ms)(milliseconds to wait=u32 50 ("毫秒倍数")) -> ()  [unwired: 1 out]
              n422 = local read "中间位置间隙"() -> (w792:dbl)
              n423 = local read "齿条推拉力(N)"() -> (w799:dbl)
              n424 = call "PCI1240电动缸读取位置.vi"("AxisHandle IN"=w805) -> ("位置"=w804:dbl)  [unwired: 9 in, 1 out]
              n425 = Subtract(x=w787, y=w806) -> (x-y=w807:dbl)
              n426 = Subtract(x=w804, y=w803) -> (x-y=w785:dbl)
              n427 = Add(x=w807, y=w792) -> (x+y=w794:dbl)
              n428 = Multiply(x=w785, y=1.12) -> (x*y=w783:dbl)
              n429 = Less Or Equal?(x=w799, y=-500.0) -> (x <= y?=w796:bool)
              n430 = Build Array (concatenate) ("创建数组")(w810, w783) -> (w781:dbl[])
              n431 = Build Array (concatenate) ("创建数组")(w801, w799) -> (w800:dbl[])
              n432 = Equal To 0?(x=w793) -> (x = 0?=w797:bool)
              n433 = Build Array (concatenate) ("创建数组")(w809, w794) -> (w808:dbl[])
              n434 = Bundle ("捆绑")(w781, w800) -> (w802:cluster{dbl[], dbl[]})  [unwired: 1 in]
              n435 = Or(x=w797, y=w796) -> (x .or. y?=w795:bool)
              n436 = Bundle ("捆绑")(w781, w808) -> (w782:cluster{dbl[], dbl[]})  [unwired: 1 in]
              n437 = Build Array ("创建数组")(w782, w802) -> (w780:cluster{dbl[], dbl[]}[])
              n438 = Less Or Equal?(x=w787, y=0.0) -> (x <= y?=w791:bool)
              n439 = Greater Or Equal?(x=w787, y=4.0) -> (x >= y?=w790:bool)
              n440 = Or(x=w790, y=w791) -> (x .or. y?=w786:bool)
              n441 = local write "行程跳动曲线"(w780) -> ()
              n442 = property on="间隙位移(mm)" class="DigNum (严格)"("Blinking"=w786) -> ()  [unwired: 2 in, 2 out]
            }
          }
          frame #17 {
            n443 = local write "电动缸速度(mm/s)"(1.0 ("电动缸速度(mm/s)")) -> ()
          }
          frame #18 {
            n444 = while {
              tunnel: w828 -> [w838]
              stop <- w837 stop-if-true
              n445 = Wait Until Next ms Multiple(millisecond multiple=u32 50 ("毫秒倍数")) -> ()  [unwired: 1 out]
              n446 = call "PCI1240电动缸位置模式 .vi"("Distance"=118.0, "AxisHandle IN"=w838) -> ("AbsSuccess"=w837:bool)  [unwired: 8 in, 1 out]
            }
          }
          frame #19 {
            n447 = while {
              shift-right: [w855] -> w852
              shift-left: w844 -> [w884]
              shift-right: [w882] -> w853
              shift-left: w845 -> [w883]
              tunnel: w843 -> [w879]
              tunnel: [w879] -> w851
              tunnel: w842 -> [w877]
              shift-right: [w874] -> w850
              shift-left: w841 -> [w875]
              stop <- w869 stop-if-true
              n448 = local read "间隙位移(mm)"() -> (w861:dbl)
              n449 = call <userlib>:"Acm_AxGetCmdVelocity.vi"("AxisHandle"=w879) -> ("Velocity"=w867:dbl)  [unwired: 1 in, 3 out]
              n450 = local read "基准位移"() -> (w880:dbl)
              n451 = Wait (ms)(milliseconds to wait=u32 50 ("毫秒倍数")) -> ()  [unwired: 1 out]
              n452 = local read "中间位置间隙"() -> (w866:dbl)
              n453 = local read "齿条推拉力(N)"() -> (w873:dbl)
              n454 = call "PCI1240电动缸读取位置.vi"("AxisHandle IN"=w879) -> ("位置"=w878:dbl)  [unwired: 9 in, 1 out]
              n455 = Subtract(x=w861, y=w880) -> (x-y=w881:dbl)
              n456 = Subtract(x=w878, y=w877) -> (x-y=w859:dbl)
              n457 = Add(x=w881, y=w866) -> (x+y=w868:dbl)
              n458 = Multiply(x=w859, y=1.12) -> (x*y=w857:dbl)
              n459 = Less Or Equal?(x=w873, y=-500.0) -> (x <= y?=w870:bool)
              n460 = Build Array (concatenate) ("创建数组")(w884, w857) -> (w855:dbl[])
              n461 = Build Array (concatenate) ("创建数组")(w875, w873) -> (w874:dbl[])
              n462 = Equal To 0?(x=w867) -> (x = 0?=w871:bool)
              n463 = Build Array (concatenate) ("创建数组")(w883, w868) -> (w882:dbl[])
              n464 = Bundle ("捆绑")(w855, w874) -> (w876:cluster{dbl[], dbl[]})  [unwired: 1 in]
              n465 = Or(x=w871, y=w870) -> (x .or. y?=w869:bool)
              n466 = Bundle ("捆绑")(w855, w882) -> (w856:cluster{dbl[], dbl[]})  [unwired: 1 in]
              n467 = Build Array ("创建数组")(w856, w876) -> (w854:cluster{dbl[], dbl[]}[])
              n468 = Less Or Equal?(x=w861, y=0.0) -> (x <= y?=w865:bool)
              n469 = Greater Or Equal?(x=w861, y=4.0) -> (x >= y?=w864:bool)
              n470 = Or(x=w864, y=w865) -> (x .or. y?=w860:bool)
              n471 = local write "行程跳动曲线"(w854) -> ()
              n472 = property on="间隙位移(mm)" class="DigNum (严格)"("Blinking"=w860) -> ()  [unwired: 2 in, 2 out]
            }
          }
          frame #20 {
            n473 = while {
              tunnel: w896 -> [w903]
              tunnel: [w902] -> _
              stop <- w901 stop-if-true
              n474 = call "PCI1220U停止.vi"("AxisHandle IN"=w903) -> ("完成"=w901:bool, "AxisHandle OUT"=w902:u32)  [unwired: 9 in]
              n475 = Wait (ms)(milliseconds to wait=u32 50 ("毫秒倍数")) -> ()  [unwired: 1 out]
            }
            n476 = Array Max & Min(array=w891) -> (max value=w895:dbl, min value=w894:dbl)  [unwired: 2 out]
            n477 = Absolute Value(x=w895) -> (abs(x)=w893:dbl)
            n478 = Absolute Value(x=w894) -> (abs(x)=w892:dbl)
            n479 = local write "右全行程间隙"(w892) -> ()
            n480 = local write "左全行程间隙"(w893) -> ()
          }
          frame #21 {
            n481 = local read "全行程180°外间隙标准(mm)"() -> (w939:dbl)
            n482 = local read "全行程180°外间隙标准(mm)"() -> (w919:dbl)
            n483 = Split 1D Array(array=w945, index=w944) -> (second subarray=w943:dbl[])  [unwired: 1 out]
            n484 = local read "全行程180°内间隙标准(mm)"() -> (w920:dbl)
            n485 = Array Max & Min(array=w935) -> (max value=w934:dbl, min value=w933:dbl)  [unwired: 2 out]
            n486 = local read "总行程标准(mm)"() -> (w914:dbl)
            n487 = call "功能计算.vi"("扭矩数组"=w943) -> ("扭差"=w930:dbl, "平均扭矩"=w942:dbl, "峰值扭矩"=w931:dbl)  [unwired: 7 in, 1 out]
            n488 = Split 1D Array(array=w923, index=w922) -> (second subarray=w921:dbl[])  [unwired: 1 out]
            n489 = Subtract(x=w934, y=w933) -> (x-y=w925:dbl)
            n490 = Subtract(x=w925, y="机械间隙值") -> (x-y=w906:dbl)
            n491 = local write "总行程(mm)"(w906) -> ()
            n492 = local write "右最大轴向力(N)"(w931) -> ()
            n493 = Greater?(x=w941, y=w939) -> (0:w927:bool)
            n494 = call "间隙计算.vi"("扭矩数组"=w921) -> ("峰值间隙1"=w938:dbl, "峰值间隙2"=w937:dbl)  [unwired: 6 in, 3 out]
            n495 = Greater?(x=w940, y=w939) -> (0:w926:bool)
            n496 = local write "右轴向力波动(N)"(w930) -> ()
            n497 = local read "总行程最大值"() -> (w915:dbl)
            n498 = In Range and Coerce "判定范围并强制转换"(upper limit=w915, x=w906, lower limit=w914) -> (In Range?=w912:bool)  [unwired: 1 out]
            n499 = Less?(x=w937, y=w919) -> (x < y?=w913:bool)
            n500 = Less?(x=w938, y=w920) -> (x < y?=w936:bool)
            n501 = local write "右平均轴向力(N)"(w942) -> ()
            n502 = local write "右180°外全行程间隙"(w937) -> ()
            n503 = local read "总圈数最大值"() -> (w916:dbl)
            n504 = local write "右180°内全行程间隙"(w938) -> ()
            n505 = property on="左全行程间隙" class="DigNum (严格)"("Blinking"=w927) -> ()  [unwired: 2 in, 2 out]
            n506 = property on="右全行程间隙" class="DigNum (严格)"("Blinking"=w926) -> ()  [unwired: 2 in, 2 out]
            n507 = Divide(x=w906, y=46.996) -> (x/y=w918:dbl)
            n508 = Not(x=w936) -> (.not. x?=w908:bool)
            n509 = Not(x=w913) -> (.not. x?=w907:bool)
            n510 = property on="右180°外全行程间隙" class="DigNum (严格)"("Blinking"=w907) -> ()  [unwired: 2 in, 2 out]
            n511 = local read "总圈数标准"() -> (w917:dbl)
            n512 = In Range and Coerce(upper limit=w916, x=w918, lower limit=w917) -> (In Range?=w911:bool)  [unwired: 1 out]
            n513 = Not(x=w912) -> (.not. x?=w910:bool)
            n514 = local write "总圈数"(w918) -> ()
            n515 = Not(x=w911) -> (.not. x?=w909:bool)
            n516 = property on="总行程(mm)" class="DigNum (严格)"("Blinking"=w910) -> ()  [unwired: 2 in, 2 out]
            n517 = property on="右180°内全行程间隙" class="DigNum (严格)"("Blinking"=w908) -> ()  [unwired: 2 in, 2 out]
            n518 = property on="总圈数" class="DigNum (严格)"("Blinking"=w909) -> ()  [unwired: 2 in, 2 out]
            "轴向力X" <- w935
            "轴向力Y" <- w945
          }
          frame #22 {
            n519 = local read "最大轴向力标准(N)"() -> (w961:dbl)
            n520 = local read "转向器中心"() -> (w966:dbl)
            n521 = local read "平均轴向力MAX(N)"() -> (w959:dbl)
            n522 = local read "轴向力标准(N)"() -> (w960:dbl)
            n523 = local read "力波动标准(N)"() -> (w958:dbl)
            n524 = call "判断.vi"("y 3"=w958, "y2-2"=w959, "y2-1"=w960, "y"=w961, "x 3"=w962, "x 2"=w969, "x"=w965) -> ("非x? 3"=w963:bool, "非x? 2"=w964:bool, "非x?"=w953:bool)  [unwired: 2 in]
            n525 = local write "电动缸速度(mm/s)"(15.0 ("电动缸速度(mm/s)")) -> ()
            n526 = property on="右最大轴向力(N)" class="DigNum (严格)"("Blinking"=w953) -> ()  [unwired: 2 in, 2 out]
            n527 = property on="右平均轴向力(N)" class="DigNum (严格)"("Blinking"=w964) -> ()  [unwired: 2 in, 2 out]
            n528 = Add(x=w966, y=-10.0) -> (x+y=w967:dbl)
          }
          frame #23 {
            n529 = Compound Arithmetic op=OR(w977, w984, w983, w982, w975, w974, w978, w981, w980, w976, w973, w972) -> (w979:bool)
            n530 = property on="右轴向力波动(N)" class="DigNum (严格)"("Blinking"=w978) -> ()  [unwired: 2 in, 2 out]
            n531 = Not(x=w979) -> (.not. x?=w985:bool)
            n532 = local write "全行程间隙及轴向力合格"(w985) -> ()
          }
          frame #24 {
            n533 = while {
              tunnel: w992 -> [w996]
              tunnel: [w994] -> w991
              tunnel: w990 -> [w993]
              stop <- w995 stop-if-true
              n534 = call "PCI1240电动缸位置模式 .vi"("Distance"=w993, "AxisHandle IN"=w996) -> ("AbsSuccess"=w995:bool, "AxisHandle OUT"=w994:u32)  [unwired: 8 in]
              n535 = Wait (ms)(milliseconds to wait=u32 50 ("毫秒倍数")) -> ()  [unwired: 1 out]
            }
          }
          frame #25 {
            n536 = while {
              tunnel: w999 -> [w1003]
              stop <- w1001 stop-if-true
              n537 = call <userlib>:"Acm_AxGetCmdVelocity.vi"("AxisHandle"=w1003) -> ("Velocity"=w1002:dbl)  [unwired: 1 in, 3 out]
              n538 = Wait Until Next ms Multiple(millisecond multiple=u32 50 ("毫秒倍数")) -> ()  [unwired: 1 out]
              n539 = Equal To 0?(x=w1002) -> (x = 0?=w1001:bool)
            }
          }
          frame #26 {
            n540 = while {
              tunnel: w1006 -> [w1010]
              tunnel: [w1008] -> w1005
              tunnel: w1004 -> [w1007]
              stop <- w1009 stop-if-true
              n541 = call "PCI1240电动缸位置模式 .vi"("Distance"=w1007, "AxisHandle IN"=w1010) -> ("AbsSuccess"=w1009:bool, "AxisHandle OUT"=w1008:u32)  [unwired: 8 in]
              n542 = Wait (ms)(milliseconds to wait=u32 50 ("毫秒倍数")) -> ()  [unwired: 1 out]
            }
          }
          frame #27 {
            n543 = while {
              tunnel: w1012 -> [w1016]
              stop <- w1014 stop-if-true
              n544 = call <userlib>:"Acm_AxGetCmdVelocity.vi"("AxisHandle"=w1016) -> ("Velocity"=w1015:dbl)  [unwired: 1 in, 3 out]
              n545 = Wait Until Next ms Multiple(millisecond multiple=u32 50 ("毫秒倍数")) -> ()  [unwired: 1 out]
              n546 = Equal To 0?(x=w1015) -> (x = 0?=w1014:bool)
            }
          }
          frame #28 {
            n547 = local read "轴向力已做次数"() -> (w1019:dbl)
            n548 = Add(x=w1019, y=1.0) -> (x+y=w1017:dbl)
            n549 = local write "轴向力已做次数"(w1017) -> ()
          }
          frame #29 {
            n550 = local read "全行程间隙及轴向力合格"() -> (w1020:bool)
            n551 = case shown="假" w1020 {
              frame False {
                n552 = Less?(x="轴向力已做次数", y="设定轴向力调整次数") -> (x < y?=w1022:bool)
                n553 = case shown="真" w1022 {
                  frame False {
                    n554 = local write "工步号"(u32 45 ("工步号")) -> ()
                  }
                  frame True {
                    n555 = local write "工步号"(u32 30 ("工步号")) -> ()
                  }
                }
              }
              frame True {
                n556 = local write "工步号"(u32 45 ("工步号")) -> ()
              }
            }
          }
        }
      }
      frame 45 {
        # "测头退回"
        n557 = flat-sequence {
          tunnel: [w1030] -> w1027
          tunnel: w1027 -> [w1037]
          frame #0 {
            n558 = local write "测头机构轴速度(mm/s)"(30.0 ("测头机构轴速度(mm/s)")) -> ()
          }
          frame #1 {
            n559 = local read "测头机构轴后退位"() -> (w1029:dbl)
            n560 = local read "测头机构电机"() -> (w1031:u32)
            n561 = while {
              tunnel: w1031 -> [w1035]
              tunnel: w1029 -> [w1034]
              tunnel: [w1033] -> w1030
              stop <- w1036 stop-if-true
              n562 = Wait Until Next ms Multiple(millisecond multiple=u32 50 ("毫秒倍数")) -> ()  [unwired: 1 out]
              n563 = call "PCI1220U进给轴位置模式.vi"("Distance"=w1034, "AxisHandle IN"=w1035) -> ("AbsSuccess"=w1036:bool, "AxisHandle OUT"=w1033:u32)  [unwired: 8 in]
            }
          }
          frame #2 {
            n564 = while {
              tunnel: w1037 -> [w1041]
              stop <- w1039 stop-if-true
              n565 = call <userlib>:"Acm_AxGetCmdVelocity.vi"("AxisHandle"=w1041) -> ("Velocity"=w1040:dbl)  [unwired: 1 in, 3 out]
              n566 = Wait Until Next ms Multiple(millisecond multiple=u32 50 ("毫秒倍数")) -> ()  [unwired: 1 out]
              n567 = Equal To 0?(x=w1040) -> (x = 0?=w1039:bool)
            }
          }
          frame #3 {
            n568 = while {
              stop <- w1042 stop-if-true
              n569 = local read "测头机构轴位置(mm)"() -> (w1044:dbl)
              n570 = Wait Until Next ms Multiple(millisecond multiple=u32 50 ("毫秒倍数")) -> ()  [unwired: 1 out]
              n571 = Less Or Equal?(x=w1044, y=35.0) -> (x <= y?=w1042:bool)
            }
          }
          frame #4 {
            n572 = local write "测头气缸左移"(TRUE ("测头气缸左移")) -> ()
            n573 = local write "测头气缸右移"(FALSE ("测头气缸右移")) -> ()
          }
          frame #5 {
            n574 = Wait Until Next ms Multiple(millisecond multiple=u32 500 ("毫秒倍数")) -> ()  [unwired: 1 out]
          }
          frame #6 {
            n575 = local write "工步号"(u32 50 ("工步号")) -> ()
          }
        }
      }
      frame 50 {
        n576 = flat-sequence {
          tunnel: [w1071] -> w1060
          tunnel: w1060 -> [w1078]
          tunnel: [w1077] -> w1058
          tunnel: w1058 -> [w1089]
          tunnel: [w1096] -> w1052
          tunnel: [w1100] -> w1053
          tunnel: w1052 -> [w1100]
          tunnel: [w1103] -> w1055
          tunnel: w1053 -> [w1102]
          tunnel: w1055 -> [w1110]
          tunnel: [w1109] -> w1054
          tunnel: w1054 -> [w1112]
          tunnel: [w1111] -> w1050
          tunnel: [w1117] -> w1051
          tunnel: w1050 -> [w1117]
          tunnel: [w1120] -> w1059
          tunnel: w1051 -> [w1119]
          tunnel: w1059 -> [w1126]
          tunnel: [w1127] -> w1057
          tunnel: w1057 -> [w1136]
          tunnel: [w1135] -> w1056
          tunnel: w1056 -> [w1146]
          frame #0 {
            n577 = local write "旋转伺服速度(°/s)"(15.0 ("调整螺塞轴速度(°/s)")) -> ()
            n578 = local write "测头机构轴速度(mm/s)"(15.0 ("调整机构轴速度(mm/s)")) -> ()
            n579 = local write "电动缸速度(mm/s)"(15.0 ("电动缸速度(mm/s)")) -> ()
            n580 = local write "夹头松开"(TRUE ("夹头松开")) -> ()
            n581 = local write "夹头夹紧"(FALSE ("夹头夹紧")) -> ()
          }
          frame #1 {
            n582 = while {
              stop <- w1066 stop-if-true
              n583 = local read "夹头夹紧位"() -> (w1069:bool)
              n584 = local read "夹头松开"() -> (w1067:bool)
              n585 = Wait Until Next ms Multiple(millisecond multiple=u32 50 ("毫秒倍数")) -> ()  [unwired: 1 out]
              n586 = Not(x=w1069) -> (.not. x?=w1068:bool)
              n587 = And(x=w1068, y=w1067) -> (x .and. y?=w1066:bool)
            }
          }
          frame #2 {
            n588 = while {
              tunnel: [w1074] -> w1071
              stop <- w1073 stop-if-true
              n589 = local read "电动缸电机"() -> (w1075:u32)
              n590 = Wait Until Next ms Multiple(millisecond multiple=u32 50 ("毫秒倍数")) -> ()  [unwired: 1 out]
              n591 = local read "齿条右极限"() -> (w1072:dbl)
              n592 = call "PCI1240电动缸位置模式 .vi"("Distance"=w1072, "AxisHandle IN"=w1075) -> ("AbsSuccess"=w1073:bool, "AxisHandle OUT"=w1074:u32)  [unwired: 8 in]
            }
          }
          frame #3 {
            n593 = while {
              tunnel: w1078 -> [w1087]
              tunnel: [w1079] -> w1077
              stop <- w1080 stop-if-true
              n594 = local read "齿条推拉力(N)"() -> (w1085:dbl)
              n595 = Wait Until Next ms Multiple(millisecond multiple=u32 50 ("毫秒倍数")) -> ()  [unwired: 1 out]
              n596 = call <userlib>:"Acm_AxGetCmdVelocity.vi"("AxisHandle"=w1087) -> ("Velocity"=w1088:dbl, "AxisHandle"=w1079:u32)  [unwired: 1 in, 2 out]
              n597 = Equal To 0?(x=w1088) -> (x = 0?=w1082:bool)
              n598 = Absolute Value(x=w1085) -> (abs(x)=w1084:dbl)
              n599 = Greater Or Equal?(x=w1084, y=1000.0) -> (x >= y?=w1081:bool)
              n600 = Or(x=w1082, y=w1081) -> (x .or. y?=w1080:bool)
            }
          }
          frame #4 {
            n601 = while {
              tunnel: w1089 -> [w1093]
              tunnel: [w1092] -> _
              stop <- w1091 stop-if-true
              n602 = call "PCI1220U停止.vi"("AxisHandle IN"=w1093) -> ("完成"=w1091:bool, "AxisHandle OUT"=w1092:u32)  [unwired: 9 in]
              n603 = Wait (ms)(milliseconds to wait=u32 50 ("毫秒倍数")) -> ()  [unwired: 1 out]
            }
          }
          frame #5 {
            n604 = local write "旋转齿条轴使能"(TRUE ("旋转齿条轴使能")) -> ()
          }
          frame #6 {
            n605 = Wait Until Next ms Multiple(millisecond multiple=u32 500 ("毫秒倍数")) -> ()  [unwired: 1 out]
          }
          frame #7 {
            n606 = local read "旋转齿条电机"() -> (w1097:u32)
            n607 = call <userlib>:"Acm_AxHome.vi"("DirMode"=u32 0, "HomeMode"=u32 11, "AxisHandle"=w1097) -> ("AxisHandle"=w1096:u32)  [unwired: 1 in, 2 out]
          }
          frame #8 {
            n608 = Wait Until Next ms Multiple(millisecond multiple=u32 100 ("毫秒倍数")) -> ()  [unwired: 1 out]
          }
          frame #9 {
            n609 = while {
              tunnel: w1102 -> [w1106]
              tunnel: [w1105] -> w1103
              stop <- w1104 stop-if-true
              n610 = call <userlib>:"Acm_AxGetCmdVelocity.vi"("AxisHandle"=w1106) -> ("Velocity"=w1108:dbl, "AxisHandle"=w1105:u32)  [unwired: 1 in, 2 out]
              n611 = Equal To 0?(x=w1108) -> (x = 0?=w1104:bool)
              n612 = Wait Until Next ms Multiple(millisecond multiple=u32 50 ("毫秒倍数")) -> ()  [unwired: 1 out]
            }
          }
          frame #10 {
            n613 = call "PCI1220U角度置零.vi"("AxisHandle IN"=w1110) -> ("AxisHandle OUT"=w1109:u32)  [unwired: 10 in]
          }
          frame #11 {
            n614 = while {
              tunnel: [w1113] -> w1111
              tunnel: w1112 -> [w1113]
              stop <- w1116 stop-if-true
              n615 = Wait Until Next ms Multiple(millisecond multiple=u32 50 ("毫秒倍数")) -> ()  [unwired: 1 out]
              n616 = call "PCI1220U扭矩轴位置模式.vi"("Distance"=15.0, "AxisHandle IN"=w1113) -> ("AbsSuccess"=w1116:bool)  [unwired: 8 in, 1 out]
            }
          }
          frame #12 {
            n617 = Wait Until Next ms Multiple(millisecond multiple=u32 100 ("毫秒倍数")) -> ()  [unwired: 1 out]
          }
          frame #13 {
            n618 = while {
              tunnel: w1119 -> [w1123]
              tunnel: [w1122] -> w1120
              stop <- w1121 stop-if-true
              n619 = call <userlib>:"Acm_AxGetCmdVelocity.vi"("AxisHandle"=w1123) -> ("Velocity"=w1125:dbl, "AxisHandle"=w1122:u32)  [unwired: 1 in, 2 out]
              n620 = Equal To 0?(x=w1125) -> (x = 0?=w1121:bool)
              n621 = Wait Until Next ms Multiple(millisecond multiple=u32 50 ("毫秒倍数")) -> ()  [unwired: 1 out]
            }
          }
          frame #14 {
            n622 = call "PCI1220U角度置零.vi"("AxisHandle IN"=w1126) -> ()  [unwired: 10 in, 1 out]
          }
          frame #15 {
            n623 = while {
              tunnel: [w1132] -> w1127
              stop <- w1131 stop-if-true
              n624 = local read "电动缸电机"() -> (w1133:u32)
              n625 = Wait Until Next ms Multiple(millisecond multiple=u32 50 ("毫秒倍数")) -> ()  [unwired: 1 out]
              n626 = local read "齿条右极限"() -> (w1130:dbl)
              n627 = Add(x=w1130, y=-10.0) -> (x+y=w1128:dbl)
              n628 = call "PCI1240电动缸位置模式 .vi"("Distance"=w1128, "AxisHandle IN"=w1133) -> ("AbsSuccess"=w1131:bool, "AxisHandle OUT"=w1132:u32)  [unwired: 8 in]
            }
          }
          frame #16 {
            n629 = while {
              tunnel: w1136 -> [w1144]
              tunnel: [w1142] -> w1135
              stop <- w1137 stop-if-true
              n630 = local read "齿条推拉力(N)"() -> (w1141:dbl)
              n631 = Wait Until Next ms Multiple(millisecond multiple=u32 50 ("毫秒倍数")) -> ()  [unwired: 1 out]
              n632 = call <userlib>:"Acm_AxGetCmdVelocity.vi"("AxisHandle"=w1144) -> ("Velocity"=w1145:dbl, "AxisHandle"=w1142:u32)  [unwired: 1 in, 2 out]
              n633 = Equal To 0?(x=w1145) -> (x = 0?=w1138:bool)
              n634 = Greater Or Equal?(x=w1141, y=300.0) -> (x >= y?=w1139:bool)
              n635 = Or(x=w1138, y=w1139) -> (x .or. y?=w1137:bool)
            }
          }
          frame #17 {
            n636 = while {
              tunnel: w1146 -> [w1150]
              tunnel: [w1149] -> _
              stop <- w1148 stop-if-true
              n637 = call "PCI1220U停止.vi"("AxisHandle IN"=w1150) -> ("完成"=w1148:bool, "AxisHandle OUT"=w1149:u32)  [unwired: 9 in]
              n638 = Wait (ms)(milliseconds to wait=u32 50 ("毫秒倍数")) -> ()  [unwired: 1 out]
            }
          }
          frame #18 {
            n639 = local write "工步号"(u32 100 ("工步号")) -> ()
          }
        }
      }
      frame 100 {
        n640 = flat-sequence {
          tunnel: [w1185] -> w1175
          tunnel: [w1183] -> w1174
          tunnel: [w1177] -> w1161
          tunnel: [w1176] -> w1159
          tunnel: w1175 -> [w1192]
          tunnel: w1174 -> [w1189]
          tunnel: ["F:\\报表存储\\" ("字符串")] -> w1173
          tunnel: [w1192] -> w1162
          tunnel: w1161 -> [w1191]
          tunnel: [w1191] -> w1160
          tunnel: w1159 -> [w1190]
          tunnel: [w1190] -> w1158
          tunnel: [w1189] -> w1157
          tunnel: w1173 -> [w1203]
          tunnel: [w1211] -> w1172
          tunnel: [w1208] -> w1171
          tunnel: [w1207] -> w1170
          tunnel: [w1206] -> w1169
          tunnel: w1162 -> [w1202]
          tunnel: w1160 -> [w1201]
          tunnel: w1158 -> [w1200]
          tunnel: w1157 -> [w1194]
          tunnel: [w1196] -> w1156
          tunnel: w1172 -> [w1218]
          tunnel: [w1219] -> w1168
          tunnel: w1171 -> [w1219]
          tunnel: w1170 -> [w1217]
          tunnel: w1169 -> [w1216]
          tunnel: [w1215] -> w1167
          tunnel: [w1214] -> w1166
          tunnel: w1156 -> [w1213]
          tunnel: [w1213] -> w1155
          tunnel: [w1226] -> w1165
          tunnel: w1168 -> [w1226]
          tunnel: w1167 -> [w1225]
          tunnel: [w1225] -> w1164
          tunnel: [w1224] -> w1163
          tunnel: w1166 -> [w1224]
          tunnel: w1155 -> [w1222]
          tunnel: [w1222] -> w1154
          tunnel: w1165 -> [w1229]
          tunnel: w1164 -> [w1237]
          tunnel: w1163 -> [w1236]
          tunnel: w1154 -> [w1228]
          tunnel: [w1228] -> w1153
          tunnel: w1153 -> [w1245]
          tunnel: [w1245] -> w1152
          tunnel: w1152 -> [w1247]
          frame #0 {
            n641 = local read "产品ID"() -> (w1184:string)
            n642 = Format Date/Time String(time format string (%c)="%Y%m%d" ("时间格式字符串(%c)")) -> (date/time string=w1178:string)  [unwired: 2 in]
            n643 = String Subset(string=w1178, offset (0)=4 ("偏移量(0)"), length (rest)=2 ("长度（剩余）")) -> (substring=w1177:string)
            n644 = String Subset(string=w1178, offset (0)=6 ("偏移量(0)"), length (rest)=2 ("长度（剩余）")) -> (substring=w1176:string)
            n645 = call <vilib>:"Trim Whitespace.vi"("string"=w1184) -> ("trimmed string"=w1183:string)  [unwired: 1 in]
            n646 = String Subset(string=w1178, offset (0)=0 ("偏移量(0)"), length (rest)=4 ("长度（剩余）")) -> (substring=w1185:string)
          }
          frame #1 {
          }
          frame #2 {
            w1195 = "\\" ("字符串")
            n647 = Concatenate Strings(w1203, w1202, w1195, w1201, w1195, w1200, w1195, w1194, w1195) -> (w1198:string)
            n648 = Concatenate Strings(w1203, w1202, w1195, w1201, w1195, w1200, w1195, w1194, w1195) -> (w1212:string)
            n649 = String To Path(string=w1212) -> (path=w1211:path)
            n650 = Concatenate Strings(w1198, w1194, "间隙曲线.JPG" ("字符串")) -> (w1209:string)
            n651 = Concatenate Strings(w1198, "轴向力曲线数组.txt" ("字符串")) -> (w1206:string)
            n652 = Concatenate Strings(w1198, "扭动曲线数组.txt" ("字符串")) -> (w1207:string)
            n653 = Concatenate Strings(w1198, w1194, "轴向力曲线.JPG" ("字符串")) -> (w1199:string)
            n654 = String To Path(string=w1209) -> (path=w1208:path)
            n655 = String To Path(string=w1199) -> (path=w1196:path)
          }
          frame #3 {
            n656 = call <vilib>:"Check if File or Folder Exists.vi"("path"=w1218) -> ("file or folder exists?"=w1220:bool)  [unwired: 8 in, 2 out]
            n657 = String To Path(string=w1216) -> (path=w1214:path)
            n658 = String To Path(string=w1217) -> (path=w1215:path)
            n659 = case shown="假" w1220 {
              tunnel: w1218 -> [w1221 _]
              frame False {
                n660 = Create Folder(path (use dialog)=w1221) -> ()  [unwired: 2 in, 3 out]
              }
              frame True {
              }
            }
          }
          frame #4 {
            n661 = local write "选项卡控件"(T1."间隙测量" ("选项卡控件")) -> ()
            n662 = Wait Until Next ms Multiple(millisecond multiple=u32 1000 ("毫秒倍数")) -> ()  [unwired: 1 out]
          }
          frame #5 {
            n663 = disable-structure shown="禁用" {
              disable-tunnel: w1229 -> [w1238 _]
              frame Disabled {
                w1242 = T2 2 items=["快速打印", "标准报表", "HTML", "双字节", "Excel"] ("report type (Quick Print)")
                w1241 = T3 1 items=["完整前面板", "前面板可见部分", "图标、说明、前面板和程序框图", "说明信息: 使用前面板", "说明信息: 作为子VI使用", "说明信息: 完整", "说明信息: 自定义"] ("contents (complete front panel)")
                n664 = Current VI's Path() -> (path=w1240:path)
                n665 = call-poly <vilib>:"Easy Print VI Panel or Documentation.vi"("report type (Quick Print)"=w1242, "contents (complete front panel)"=w1241, "VI path"=w1240) -> ("error out"=w1244:errorcluster, "report out"=w1243:refnum<class "NI_report.lvclass">)  [unwired: 1 in, 6 out]
                n666 = call-dynamic "Save Report to File.vi"("report in"=w1243, "report file path"=w1238, "error in (no error)"=w1244) -> ("error out"=→"error out 3":errorcluster)  [unwired: 2 in, 10 out]
              }
              frame Enabled {
              }
            }
            n667 = local read "间隙Y数组"() -> (w1234:dbl[])
            n668 = local read "间隙X数组"() -> (w1235:dbl[])
            n669 = local read "轴向力Y"() -> (w1232:dbl[])
            n670 = local read "轴向力X"() -> (w1233:dbl[])
            n671 = call "导出曲线数组.vi"("file path (dialog if empty)"=w1237, "数组 2"=w1234, "数组"=w1235) -> ()  [unwired: 9 in]
            n672 = call "导出曲线数组.vi"("file path (dialog if empty)"=w1236, "数组 2"=w1232, "数组"=w1233) -> ()  [unwired: 9 in]
            n673 = control-ref of="本VI"() -> (w1231:refnum<vi>)
            n674 = invoke class="VI" method="FP.Get Image"(reference=w1231) -> ("image data"=w1230:T4)  [unwired: 5 in, 5 out]
            n675 = call <vilib>:"Write JPEG File.vi"("image data"=w1230, "path to JPEG file"=w1229) -> ()  [unwired: 8 in, 2 out]
          }
          frame #6 {
            n676 = local write "选项卡控件"(T1."轴向力测量" ("选项卡控件")) -> ()
          }
          frame #7 {
            n677 = control-ref of="本VI"() -> (w1248:refnum<vi>)
            n678 = invoke class="VI" method="FP.Get Image"(reference=w1248) -> ("image data"=w1249:T4)  [unwired: 5 in, 5 out]
            n679 = call <vilib>:"Write JPEG File.vi"("image data"=w1249, "path to JPEG file"=w1247) -> ()  [unwired: 8 in, 2 out]
          }
          frame #8 {
            n680 = local read "联线按钮"() -> (w1250:bool)
            n681 = case shown="真" w1250 {
              frame False {
              }
              frame True {
                n682 = flat-sequence {
                  tunnel: [w1257] -> w1251
                  tunnel: w1251 -> [w1274]
                  frame #0 {
                    n683 = local read "全行程间隙及轴向力合格"() -> (w1252:bool)
                    n684 = local read "单点间隙合格"() -> (w1253:bool)
                    n685 = local read "左全行程间隙"() -> (w1260:dbl)
                    n686 = local read "中间位置间隙"() -> (w1263:dbl)
                    n687 = local read "FGCS"() -> (w1265:string)
                    n688 = local read "员工ID"() -> (w1270:string)
                    n689 = And(x=w1253, y=w1252) -> (x .and. y?=w1254:bool)
                    n690 = local read "KSJJ"() -> (w1267:string)
                    n691 = local read "产品ID"() -> (w1271:string)
                    n692 = Boolean To (0,1)(Boolean=w1254) -> (0, 1=w1269:i16)
                    n693 = Format Date/Time String(time format string (%c)="%Y%m%d%H%M" ("时间格式字符串(%c)")) -> (date/time string=w1266:string)  [unwired: 2 in]
                    n694 = Number To Decimal String(number=w1269, width (-)=i16 1 ("宽度(-)")) -> (decimal integer string=w1255:string)
                    n695 = Number To Fractional String(number=w1260, precision (6)=i16 3 ("精度(6)")) -> (F-format string=w1258:string)  [unwired: 2 in]
                    n696 = Number To Fractional String(number=w1263, precision (6)=i16 3 ("精度(6)")) -> (F-format string=w1259:string)  [unwired: 2 in]
                    n697 = Build Array(w1271, w1270, "1", w1255, w1267, w1266, w1265, "Q14070-Z060A", w1259, w1258) -> (w1257:string[])
                  }
                  frame #1 {
                    n698 = Wait (ms)(milliseconds to wait=u32 500 ("等待时间（毫秒）")) -> ()  [unwired: 1 out]
                    n699 = call "数据库更新.vi"("设备号"="06", "数据"=w1274) -> ()  [unwired: 13 in, 1 out]
                  }
                  frame #2 {
                  }
                }
              }
            }
          }
          frame #9 {
            n700 = local write "产品ID"("") -> ()
            n701 = local write "工步号"(u32 0 ("工步号")) -> ()
          }
        }
      }
    }
    n702 = Wait (ms)(milliseconds to wait=u32 50 ("毫秒倍数")) -> ()  [unwired: 1 out]
    n703 = local read "停止"() -> (w7:bool)
  }
  n704 = while {
    stop <- w1278 stop-if-true
    n705 = event shown="[2] \"参数修改\": 值改变" {
      selector: _ -> [_ _ _ _ _ _ _]
      dyn-events: _ -> [_ _ _ _ _ _ _]
      timeout: 500 -> [_ _ _ _ _ _ _]
      event Timeout {
        n706 = event-data() -> ()  [unwired: 3 out]
      }
      event "停止": Value Change {
        n707 = event-data() -> ()  [unwired: 6 out]
        n708 = flat-sequence {
          frame #0 {
            n709 = Wait (ms)(milliseconds to wait=u32 1000 ("毫秒倍数")) -> ()  [unwired: 1 out]
          }
          frame #1 {
            n710 = Quit LabVIEW(quit? (T)=TRUE ("停止？(T)")) -> ()
          }
        }
      }
      event "参数修改": Value Change {
        n711 = event-data() -> ()  [unwired: 6 out]
        n712 = while {
          i -> [w1330]
          stop <- w1329 stop-if-true
          n713 = local read "型号数量"() -> (w1331:i32)
          n714 = local read "参数浏览表"() -> (w1332:string[][])
          n715 = Greater Or Equal?(x=w1330, y=w1331) -> (x >= y?=w1329:bool)
          n716 = Wait Until Next ms Multiple(millisecond multiple=u32 50 ("毫秒倍数")) -> ()  [unwired: 1 out]
          n717 = Index Array(array=w1332, index (col)=w1330) -> (element=w1317:string[])  [unwired: 1 in]
          n718 = Index Array(array=w1317, index #1=0 ("索引"), index #2=2 ("索引"), index #3=3 ("索引"), index #4=4 ("索引"), index #5=5 ("索引"), index #6=6 ("索引"), index #7=7 ("索引"), index #8=8 ("索引"), index #9=9 ("索引"), index #10=10 ("索引"), index #11=11 ("索引"), index #12=12 ("索引"), index #13=13 ("索引"), index #14=14 ("索引"), index #15=15 ("索引"), index #16=16 ("索引"), index #17=17 ("索引"), index #18=18 ("索引"), index #19=19 ("索引"), index #20=20 ("索引")) -> (element #1=w1284:string, element #2=w1313:string, element #3=w1312:string, element #4=w1311:string, element #5=w1310:string, element #6=w1309:string, element #7=w1308:string, element #8=w1307:string, element #9=w1306:string, element #10=w1305:string, element #11=w1304:string, element #12=w1299:string, element #13=w1298:string, element #14=w1297:string, element #15=w1296:string, element #16=w1295:string, element #17=w1290:string, element #18=w1289:string, element #19=w1288:string, element #20=w1283:string)
          n719 = call "创建文本"("测头机构轴移动速度"=w1313, "测头机构轴检测位"=w1312, "测头机构轴待检位"=w1311, "测头机构轴后退位"=w1310, "齿条移动速度"=w1309, "齿条左极限"=w1308, "齿条右极限"=w1307, "旋转齿条轴找帽转速"=w1306, "旋转齿条轴测量转速"=w1305, "测量点扭矩"=w1304, "总行程最大值"=w1298, "总行程最小值"=w1299, "最大轴向力"=w1297, "轴向力波动"=w1296, "平均轴向力最小值"=w1295, "平均轴向力最大值"=w1290, "总圈数最小值"=w1289, "总圈数最大值"=w1288, "中间位置"=w1283, "产品型号"=w1284) -> ("Result"=w1303:string)  [unwired: 6 in, 1 out]
          n720 = local read "ADODB._Connection Out 2"() -> (w1302:refnum<k7>)
          n721 = call "SQL Execute.vi"("Command Text"=w1303, "ADODB._Connection In"=w1302) -> ("error out"=w1315:errorcluster, "ADODB._Connection Out"=w1316:refnum<k7>)  [unwired: 6 in, 2 out]
          n722 = call "ADO Connection Close.vi"("error in (no error)"=w1315, "ADODB._Connection In"=w1316) -> ("error out"=→"error out":errorcluster)  [unwired: 8 in, 1 out]
        }
      }
      event "参数查询": Value Change {
        n723 = event-data() -> ()  [unwired: 6 out]
        n724 = flat-sequence {
          tunnel: [w1345] -> w1338
          tunnel: [w1344] -> w1337
          tunnel: [w1343] -> w1334
          tunnel: w1338 -> [w1349]
          tunnel: w1337 -> [w1351]
          tunnel: [w1351] -> w1336
          tunnel: [w1350] -> w1335
          tunnel: w1334 -> [w1350]
          tunnel: w1336 -> [_]
          tunnel: w1335 -> [_]
          frame #0 {
            n725 = call-poly <vilib>:"Read From Spreadsheet File.vi"("file path (dialog if empty)"=path "D:/Q14070-Z060人机界面/参数/参数项.txt") -> ("first row"=w1339:string[])  [unwired: 6 in, 4 out]
            n726 = property on="参数浏览表" class="Tbl (严格)"("Row Headers[]"=w1339) -> ()  [unwired: 2 in, 2 out]
          }
          frame #1 {
            n727 = local read "ADODB._Connection Out 2"() -> (w1342:refnum<k7>)
            n728 = call "SQL Execute.vi"("Command Text"="SELECT * FROM 测试参数表;", "ADODB._Connection In"=w1342) -> ("error out"=w1343:errorcluster, "Data"=w1347:string[][], "ADODB._Connection Out"=w1344:refnum<k7>)  [unwired: 6 in, 1 out]
            n729 = Transpose 2D Array(2D array=w1347) -> (transposed array=w1345:string[][])
            n730 = Index Array(array=w1345, index (row)=0 ("索引 (行)")) -> (element=w1346:string[])  [unwired: 1 in]
            n731 = property on="参数浏览表" class="Tbl (严格)"("Column Headers[]"=w1346) -> ()  [unwired: 2 in, 2 out]
          }
          frame #2 {
            n732 = local write "参数浏览表"(w1349) -> ()
          }
          frame #3 {
          }
        }
      }
      event "传感器参数保存": Value Change {
        n733 = event-data() -> ()  [unwired: 6 out]
        n734 = flat-sequence {
          tunnel: [w1377] -> w1374
          tunnel: [w1376] -> w1373
          tunnel: [w1375] -> w1372
          tunnel: [w1383] -> w1371
          tunnel: w1374 -> [w1383]
          tunnel: [w1382] -> w1370
          tunnel: w1373 -> [w1382]
          tunnel: [w1381] -> w1369
          tunnel: w1372 -> [w1381]
          tunnel: [w1380] -> w1368
          tunnel: [w1379] -> w1367
          tunnel: [w1378] -> w1366
          tunnel: [w1384] -> w1365
          tunnel: [w1390] -> w1364
          tunnel: w1371 -> [w1390]
          tunnel: [w1389] -> w1363
          tunnel: w1370 -> [w1389]
          tunnel: w1369 -> [w1388]
          tunnel: [w1388] -> w1362
          tunnel: [w1387] -> w1361
          tunnel: w1368 -> [w1387]
          tunnel: [w1386] -> w1360
          tunnel: w1367 -> [w1386]
          tunnel: [w1385] -> w1359
          tunnel: w1366 -> [w1385]
          tunnel: w1365 -> [w1409]
          tunnel: [w1409] -> w1358
          tunnel: w1364 -> [w1408]
          tunnel: w1363 -> [w1401]
          tunnel: w1362 -> [w1400]
          tunnel: w1361 -> [w1394]
          tunnel: w1360 -> [w1393]
          tunnel: w1359 -> [w1399]
          tunnel: [w1398] -> w1357
          tunnel: [w1397] -> w1356
          tunnel: [w1396] -> w1355
          tunnel: [w1392] -> w1354
          tunnel: [w1391] -> w1353
          tunnel: [w1395] -> w1352
          tunnel: w1358 -> [w1417]
          tunnel: w1357 -> [w1416]
          tunnel: w1356 -> [w1415]
          tunnel: w1355 -> [w1414]
          tunnel: w1354 -> [w1413]
          tunnel: w1353 -> [w1412]
          tunnel: w1352 -> [w1411]
          frame #0 {
            n735 = local read "齿条推拉力零点偏移"() -> (w1376:dbl)
            n736 = local read "间隙位移零点偏移"() -> (w1377:dbl)
            n737 = local read "齿条扭矩零点偏移"() -> (w1375:dbl)
          }
          frame #1 {
            n738 = local read "齿条推拉力比例偏移"() -> (w1379:dbl)
            n739 = local read "间隙位移比例偏移"() -> (w1380:dbl)
            n740 = local read "齿条扭矩比例偏移"() -> (w1378:dbl)
          }
          frame #2 {
            n741 = local read "ADODB._Connection Out 2"() -> (w1384:refnum<k7>)
          }
          frame #3 {
            n742 = Number To Fractional String(number=w1408, precision (6)=i16 2 ("精度(6)")) -> (F-format string=w1398:string)  [unwired: 2 in]
            n743 = Number To Fractional String(number=w1400, precision (6)=i16 2 ("精度(6)")) -> (F-format string=w1396:string)  [unwired: 2 in]
            n744 = Number To Fractional String(number=w1399, precision (6)=i16 2 ("精度(6)")) -> (F-format string=w1395:string)  [unwired: 2 in]
            n745 = Number To Fractional String(number=w1401, precision (6)=i16 2 ("精度(6)")) -> (F-format string=w1397:string)  [unwired: 2 in]
            n746 = Number To Fractional String(number=w1394, precision (6)=i16 2 ("精度(6)")) -> (F-format string=w1392:string)  [unwired: 2 in]
            n747 = Number To Fractional String(number=w1393, precision (6)=i16 2 ("精度(6)")) -> (F-format string=w1391:string)  [unwired: 2 in]
          }
          frame #4 {
            n748 = call "创建文本3"("4"=w1413, "6"=w1411, "1"=w1416, "2"=w1415, "3"=w1414, "5"=w1412) -> ("Result"=w1418:string)  [unwired: 8 in, 1 out]
            n749 = call "SQL Execute.vi"("Command Text"=w1418, "ADODB._Connection In"=w1417) -> ("error out"=→"error out 4":errorcluster)  [unwired: 6 in, 3 out]
          }
        }
      }
      event "产品ID": Value Change {
        n750 = event-data() -> ()  [unwired: 7 out]
        n751 = Format Date/Time String(time format string (%c)="%Y%m%d%H%M" ("时间格式字符串(%c)")) -> (date/time string=w1419:string)  [unwired: 2 in]
        n752 = local write "KSJJ"(w1419) -> ()
      }
      event "电动缸回零": Mouse Down {
        n753 = event-data() -> ()  [unwired: 6 out]
        n754 = stacked-sequence {
          frame #0 {
            n755 = flat-sequence {
              tunnel: [w1439] -> w1428
              tunnel: [w1432] -> w1425
              tunnel: w1428 -> [w1442]
              tunnel: [w1442] -> w1427
              tunnel: [w1440] -> w1426
              tunnel: w1425 -> [w1440]
              tunnel: w1427 -> [w1444]
              tunnel: [w1444] -> w1429
              tunnel: w1426 -> [w1443]
              tunnel: [w1443] -> w1424
              tunnel: w1429 -> [w1455]
              tunnel: w1424 -> [w1454]
              tunnel: [w1453] -> w1423
              tunnel: w1423 -> [w1457]
              tunnel: [w1456] -> w1422
              tunnel: w1422 -> [w1465]
              frame #0 {
                n756 = local write "电动缸速度(mm/s)"(15.0 ("电动缸速度(mm/s)")) -> ()
                n757 = local write "测头机构轴速度(mm/s)"(10.0 ("电动缸速度(mm/s)")) -> ()
              }
              frame #1 {
                n758 = local read "测头机构电机"() -> (w1436:u32)
                n759 = local read "电动缸电机"() -> (w1433:u32)
                n760 = call <userlib>:"Acm_AxHome.vi"("DirMode"=u32 0, "HomeMode"=u32 11, "AxisHandle"=w1436) -> ("AxisHandle"=w1439:u32)  [unwired: 1 in, 2 out]
                n761 = call <userlib>:"Acm_AxHome.vi"("DirMode"=u32 1, "HomeMode"=u32 11, "AxisHandle"=w1433) -> ("AxisHandle"=w1432:u32)  [unwired: 1 in, 2 out]
              }
              frame #2 {
                n762 = Wait Until Next ms Multiple(millisecond multiple=u32 100 ("毫秒倍数")) -> ()  [unwired: 1 out]
              }
              frame #3 {
                n763 = while {
                  tunnel: w1444 -> [w1452]
                  stop <- w1450 stop-if-true
                  n764 = call <userlib>:"Acm_AxGetCmdVelocity.vi"("AxisHandle"=w1452) -> ("Velocity"=w1451:dbl)  [unwired: 1 in, 3 out]
                  n765 = Wait Until Next ms Multiple(millisecond multiple=u32 50 ("毫秒倍数")) -> ()  [unwired: 1 out]
                  n766 = Equal To 0?(x=w1451) -> (x = 0?=w1450:bool)
                }
                n767 = while {
                  tunnel: w1443 -> [w1448]
                  stop <- w1446 stop-if-true
                  n768 = call <userlib>:"Acm_AxGetCmdVelocity.vi"("AxisHandle"=w1448) -> ("Velocity"=w1447:dbl)  [unwired: 1 in, 3 out]
                  n769 = Wait Until Next ms Multiple(millisecond multiple=u32 50 ("毫秒倍数")) -> ()  [unwired: 1 out]
                  n770 = Equal To 0?(x=w1447) -> (x = 0?=w1446:bool)
                }
              }
              frame #4 {
                n771 = call "PCI1220U角度置零.vi"("AxisHandle IN"=w1455) -> ()  [unwired: 10 in, 1 out]
                n772 = call "PCI1220U角度置零.vi"("AxisHandle IN"=w1454) -> ("AxisHandle OUT"=w1453:u32)  [unwired: 10 in]
              }
              frame #5 {
                n773 = while {
                  tunnel: [w1463] -> w1456
                  tunnel: w1457 -> [w1458]
                  stop <- w1462 stop-if-true
                  n774 = Wait Until Next ms Multiple(millisecond multiple=u32 50 ("毫秒倍数")) -> ()  [unwired: 1 out]
                  n775 = local read "齿条右极限"() -> (w1461:dbl)
                  n776 = Add(x=w1461, y=-10.0) -> (x+y=w1459:dbl)
                  n777 = call "PCI1240电动缸位置模式 .vi"("Distance"=w1459, "AxisHandle IN"=w1458) -> ("AbsSuccess"=w1462:bool, "AxisHandle OUT"=w1463:u32)  [unwired: 8 in]
                }
              }
              frame #6 {
                n778 = while {
                  tunnel: w1465 -> [w1469]
                  stop <- w1467 stop-if-true
                  n779 = call <userlib>:"Acm_AxGetCmdVelocity.vi"("AxisHandle"=w1469) -> ("Velocity"=w1468:dbl)  [unwired: 1 in, 3 out]
                  n780 = Wait Until Next ms Multiple(millisecond multiple=u32 50 ("毫秒倍数")) -> ()  [unwired: 1 out]
                  n781 = Equal To 0?(x=w1468) -> (x = 0?=w1467:bool)
                }
              }
            }
          }
          frame #1 {
            n782 = flat-sequence {
              tunnel: [w1481] -> w1476
              tunnel: w1476 -> [w1483]
              tunnel: [w1483] -> w1475
              tunnel: w1475 -> [w1484]
              tunnel: [w1484] -> w1474
              tunnel: w1474 -> [w1490]
              tunnel: [w1489] -> w1471
              tunnel: w1471 -> [w1492]
              tunnel: [w1492] -> w1470
              tunnel: w1470 -> [w1494]
              tunnel: [w1493] -> w1473
              tunnel: w1473 -> [w1500]
              tunnel: [w1500] -> w1472
              tunnel: w1472 -> [w1505]
              frame #0 {
                n783 = local write "旋转伺服速度(°/s)"(5.0 ("电动缸速度(mm/s)")) -> ()
              }
              frame #1 {
                n784 = local read "旋转齿条电机"() -> (w1478:u32)
                n785 = call <userlib>:"Acm_AxHome.vi"("DirMode"=u32 0, "HomeMode"=u32 11, "AxisHandle"=w1478) -> ("AxisHandle"=w1481:u32)  [unwired: 1 in, 2 out]
              }
              frame #2 {
                n786 = Wait Until Next ms Multiple(millisecond multiple=u32 100 ("毫秒倍数")) -> ()  [unwired: 1 out]
              }
              frame #3 {
                n787 = while {
                  tunnel: w1484 -> [w1488]
                  stop <- w1486 stop-if-true
                  n788 = call <userlib>:"Acm_AxGetCmdVelocity.vi"("AxisHandle"=w1488) -> ("Velocity"=w1487:dbl)  [unwired: 1 in, 3 out]
                  n789 = Wait Until Next ms Multiple(millisecond multiple=u32 50 ("毫秒倍数")) -> ()  [unwired: 1 out]
                  n790 = Equal To 0?(x=w1487) -> (x = 0?=w1486:bool)
                }
              }
              frame #4 {
                n791 = call "PCI1220U角度置零.vi"("AxisHandle IN"=w1490) -> ("AxisHandle OUT"=w1489:u32)  [unwired: 10 in]
              }
              frame #5 {
                n792 = Wait (ms)(milliseconds to wait=u32 100 ("等待时间（毫秒）")) -> ()  [unwired: 1 out]
              }
              frame #6 {
                n793 = while {
                  tunnel: [w1498] -> w1493
                  tunnel: w1494 -> [w1495]
                  stop <- w1497 stop-if-true
                  n794 = Wait Until Next ms Multiple(millisecond multiple=u32 50 ("毫秒倍数")) -> ()  [unwired: 1 out]
                  n795 = call "PCI1220U扭矩轴位置模式.vi"("Distance"=15.0, "AxisHandle IN"=w1495) -> ("AbsSuccess"=w1497:bool, "AxisHandle OUT"=w1498:u32)  [unwired: 8 in]
                }
              }
              frame #7 {
                n796 = while {
                  tunnel: w1500 -> [w1503]
                  stop <- w1501 stop-if-true
                  n797 = call <userlib>:"Acm_AxGetCmdVelocity.vi"("AxisHandle"=w1503) -> ("Velocity"=w1504:dbl)  [unwired: 1 in, 3 out]
                  n798 = Wait Until Next ms Multiple(millisecond multiple=u32 50 ("毫秒倍数")) -> ()  [unwired: 1 out]
                  n799 = Equal To 0?(x=w1504) -> (x = 0?=w1501:bool)
                }
              }
              frame #8 {
                n800 = call "PCI1220U角度置零.vi"("AxisHandle IN"=w1505) -> ()  [unwired: 10 in, 1 out]
              }
            }
          }
          frame #2 {
            n801 = flat-sequence {
              frame #0 {
                n802 = while {
                  stop <- w1509 stop-if-true
                  n803 = local read "电动缸回零"() -> (w1510:bool)
                  n804 = local write "回零完成"(TRUE ("回零完成")) -> ()
                  n805 = local write "电动缸回零"(FALSE ("电动缸回零")) -> ()
                  n806 = Wait Until Next ms Multiple(millisecond multiple=u32 50 ("毫秒倍数")) -> ()  [unwired: 1 out]
                  n807 = Not(x=w1510) -> (.not. x?=w1509:bool)
                }
              }
            }
          }
        }
        n808 = Wait Until Next ms Multiple(millisecond multiple=u32 50 ("毫秒倍数")) -> ()  [unwired: 1 out]
      }
    }
    n809 = Wait (ms)(milliseconds to wait=u32 50 ("毫秒倍数")) -> ()  [unwired: 1 out]
    n810 = local read "停止"() -> (w1278:bool)
  }
  n811 = call "PCI1240电动缸位置模式 .vi"() -> ()  [unwired: 10 in, 2 out]
  n812 = while {
    stop <- w1512 stop-if-true
    n813 = stacked-sequence {
      frame #0 {
        n814 = flat-sequence {
          frame #0 {
          }
          frame #1 {
            n815 = First Call?() -> (First Call?: T/F=w1513:bool)
            n816 = case shown="真" w1513 {
              frame False {
              }
              frame True {
                n817 = call "员工管理测试程序.vi"() -> ("员工姓名"=w1515:string, "员工ID"=w1514:string)  [unwired: 10 in]
                n818 = local write "员工ID"(w1514) -> ()
                n819 = local write "员工姓名"(w1515) -> ()
              }
            }
          }
          frame #2 {
          }
          frame #3 {
          }
          frame #4 {
          }
          frame #5 {
          }
          frame #6 {
          }
        }
      }
      frame #1 {
        n820 = flat-sequence {
          frame #0 {
            n821 = property on="型号选择" class="Ring (严格)"() -> ("RingText.Text"=w1516:string)  [unwired: 2 in, 2 out]
            n822 = case shown="\"J706\"" w1516 {
              frame "J706" {
                w1517 = FALSE ("可见")
                w1518 = TRUE ("可见")
                n823 = property on="左180°内全行程间隙" class="DigNum (严格)"("Visible"=w1518) -> ()  [unwired: 2 in, 2 out]
                n824 = property on="左180°外全行程间隙" class="DigNum (严格)"("Visible"=w1518) -> ()  [unwired: 2 in, 2 out]
                n825 = property on="右180°外全行程间隙" class="DigNum (严格)"("Visible"=w1518) -> ()  [unwired: 2 in, 2 out]
                n826 = property on="右180°内全行程间隙" class="DigNum (严格)"("Visible"=w1518) -> ()  [unwired: 2 in, 2 out]
                n827 = property on="左全行程间隙" class="DigNum (严格)"("Visible"=w1517) -> ()  [unwired: 2 in, 2 out]
                n828 = property on="右全行程间隙" class="DigNum (严格)"("Visible"=w1517) -> ()  [unwired: 2 in, 2 out]
              }
              frame "J728" {
                w1519 = FALSE ("可见")
                w1520 = TRUE ("可见")
                n829 = property on="左180°内全行程间隙" class="DigNum (严格)"("Visible"=w1520) -> ()  [unwired: 2 in, 2 out]
                n830 = property on="左180°外全行程间隙" class="DigNum (严格)"("Visible"=w1520) -> ()  [unwired: 2 in, 2 out]
                n831 = property on="右180°外全行程间隙" class="DigNum (严格)"("Visible"=w1520) -> ()  [unwired: 2 in, 2 out]
                n832 = property on="右180°内全行程间隙" class="DigNum (严格)"("Visible"=w1520) -> ()  [unwired: 2 in, 2 out]
                n833 = property on="左全行程间隙" class="DigNum (严格)"("Visible"=w1519) -> ()  [unwired: 2 in, 2 out]
                n834 = property on="右全行程间隙" class="DigNum (严格)"("Visible"=w1519) -> ()  [unwired: 2 in, 2 out]
              }
              frame "J709", Default {
                w1521 = TRUE ("可见")
                w1522 = FALSE ("可见")
                n835 = property on="左180°内全行程间隙" class="DigNum (严格)"("Visible"=w1522) -> ()  [unwired: 2 in, 2 out]
                n836 = property on="左180°外全行程间隙" class="DigNum (严格)"("Visible"=w1522) -> ()  [unwired: 2 in, 2 out]
                n837 = property on="右180°外全行程间隙" class="DigNum (严格)"("Visible"=w1522) -> ()  [unwired: 2 in, 2 out]
                n838 = property on="右180°内全行程间隙" class="DigNum (严格)"("Visible"=w1522) -> ()  [unwired: 2 in, 2 out]
                n839 = property on="左全行程间隙" class="DigNum (严格)"("Visible"=w1521) -> ()  [unwired: 2 in, 2 out]
                n840 = property on="右全行程间隙" class="DigNum (严格)"("Visible"=w1521) -> ()  [unwired: 2 in, 2 out]
              }
            }
          }
          frame #1 {
            (unwired) string[] ["I急停按钮", "I自动旋钮", "I启动按钮", "I备用按钮", "I复位按钮", "I上阻挡器放行", "I下阻挡器放行", "I进支线按钮"] ("I0说明")
            (unwired) string[] ["I出支线按钮", "I主线顶升按钮", "I主线下降按钮", "I支线顶升按钮", "I支线下降按钮", "I气压报警", "未使用", "未使用"] ("I0说明")
            n841 = local read "间隙位移(mm)"() -> (w1525:dbl)
            n842 = Greater Or Equal?(x=w1525, y=7.0) -> (x >= y?=w1523:bool)
            n843 = case shown="真" w1523 {
              frame False {
              }
              frame True {
                n844 = local write "测头机构轴使能"(FALSE ("测头机构轴使能")) -> ()
              }
            }
          }
          frame #2 {
            (unwired) string[] ["I电动缸SRDY", "I电动缸ZSPD", "I电动缸ALRM", "I间隙进给SRDY", "I间隙进给ZSPD", "I间隙进给ALRM", "I间隙旋转SRPD", "I间隙旋转ZSPD"] ("I0说明")
            n845 = local read "测头机构轴位置(mm)"() -> (w1529:dbl)
            n846 = Greater Or Equal?(x=w1529, y=90.0) -> (x >= y?=w1527:bool)
            n847 = case shown="假" w1527 {
              frame False {
                w1530 = T5."Enabled" ("禁用")
                n848 = property on="测头气缸左移" class="Bool (严格)"("DisabledEnum"=w1530) -> ()  [unwired: 2 in, 2 out]
                n849 = property on="测头气缸右移" class="Bool (严格)"("DisabledEnum"=w1530) -> ()  [unwired: 2 in, 2 out]
                n850 = property on="测头气缸左移" class="Bool"("DisabledEnum"=w1530) -> ()  [unwired: 2 in, 2 out]
                n851 = property on="测头气缸右移" class="Bool"("DisabledEnum"=w1530) -> ()  [unwired: 2 in, 2 out]
              }
              frame True {
                w1531 = T5."Disabled" ("禁用")
                w1532 = FALSE ("测头气缸右移")
                n852 = local write "测头气缸右移"(w1532) -> ()
                n853 = local write "测头气缸左移"(w1532) -> ()
                n854 = property on="测头气缸左移" class="Bool (严格)"("DisabledEnum"=w1531) -> ()  [unwired: 2 in, 2 out]
                n855 = property on="测头气缸右移" class="Bool (严格)"("DisabledEnum"=w1531) -> ()  [unwired: 2 in, 2 out]
                n856 = property on="测头气缸左移" class="Bool"("DisabledEnum"=w1531) -> ()  [unwired: 2 in, 2 out]
                n857 = property on="测头气缸右移" class="Bool"("DisabledEnum"=w1531) -> ()  [unwired: 2 in, 2 out]
              }
            }
          }
          frame #3 {
            (unwired) string[] ["I间隙旋转ALRM", "I扭矩旋转SRPD", "I扭矩旋转ZSPD", "I扭矩旋转ALRM", "I拧紧机合格", "I拧紧机不合格", "I拧紧机报警", "未使用"] ("I0说明")
          }
        }
      }
      frame #2 {
        n858 = flat-sequence {
          frame #0 {
            (unwired) string[] ["I自制气缸进位", "I自制气缸原位", "I上工位检测", "I本工位检测", "I下工位检测", "I主线顶升上位", "I主线顶升下位", "I支线顶升上位"] ("I0说明")
          }
          frame #1 {
            (unwired) string[] ["I支线顶升下位", "I支线进到位", "I支线退到位", "I位移气缸原位", "I位移气缸进位", "I拧紧机在位", "I电动缸原位", "I电动缸进位"] ("I0说明")
          }
          frame #2 {
            (unwired) string[] ["未使用", "未使用", "未使用", "未使用", "未使用", "未使用", "未使用", "未使用"] ("I0说明")
          }
          frame #3 {
            (unwired) string[] ["未使用", "未使用", "未使用", "未使用", "未使用", "未使用", "未使用", "未使用"] ("I0说明")
          }
        }
        n859 = local read "下工位测试H"() -> (w1534:bool)
        n860 = local read "下工位备料H"() -> (w1533:bool)
        n861 = local read "下工位自动H"() -> (w1535:bool)
        n862 = local write "下工位备料"(w1533) -> ()
        n863 = local write "下工位测试"(w1534) -> ()
        n864 = local write "下工位自动"(w1535) -> ()
      }
      frame #3 {
        n865 = local read "工步号"() -> (w1539:u32)
        n866 = local read "报警"() -> (w1537:dbl)
        n867 = case shown="50" w1539 {
          tunnel: [w1550 "请取胶瓶" ("工步描述") "请取扳手加力" ("工步描述") "灵敏度测试中" ("工步描述") "有油刚度测试中" ("工步描述") "点击启动按钮进行测试" ("工步描述") "电动缸前进找中" ("工步描述") "气缸右移" ("工步描述") "电动缸前进找中" ("工步描述") "找中结束开始测间隙" ("工步描述") "力特性试验中" ("工步描述") "轴向力测试中" ("工步描述") "探头气缸左移，电动缸后退" ("工步描述") "等待放行" ("工步描述") "电动缸回零" ("工步描述") "力特性试验完成" ("工步描述") "套好输出轴把手，按启动按钮，做回正力试验" ("工步描述") "回正力试验中" ("工步描述") "试验完成，将把手拉回，取下油管，按顶升按钮" ("工步描述") "拆下锁紧螺母和输入轴万向节，按顶升按钮" ("工步描述")] -> w1538
          frame 0, Default {
            n868 = local read "联线按钮"() -> (w1549:bool)
            n869 = case shown="假" w1549 {
              tunnel: ["等待工件" ("工步描述") "等待扫描条码" ("工步描述")] -> w1550
              frame False {
              }
              frame True {
              }
            }
          }
          frame 1 {
          }
          frame 2 {
          }
          frame 3 {
          }
          frame 4 {
          }
          frame 6 {
          }
          frame 7 {
          }
          frame 10 {
          }
          frame 15 {
          }
          frame 20 {
          }
          frame 30 {
          }
          frame 40 {
          }
          frame 45 {
          }
          frame 100 {
          }
          frame 50 {
          }
          frame 55 {
          }
          frame 60 {
          }
          frame 70 {
          }
          frame 80 {
          }
          frame 56 {
          }
        }
        "工步提示" <- w1538
        n870 = case shown="9" w1537 {
          tunnel: [_ "探头气缸不在原位" "操作步骤错误请取胶瓶" "操作步骤错误请加力" "急停被按下" "气压报警" "电动缸伺服报警" "旋转伺服报警" "测头伺服报警" "操作步骤错误请点标后放行"] -> w1536
          frame 0, Default {
          }
          frame 1 {
          }
          frame 2 {
          }
          frame 3 {
          }
          frame 4 {
          }
          frame 5 {
          }
          frame 6 {
          }
          frame 7 {
          }
          frame 8 {
          }
          frame 9 {
          }
        }
        n871 = local write "报警提示"(w1536) -> ()
      }
      frame #4 {
        n872 = local read "急停"() -> (w1572:bool)
        n873 = local read "红灯"() -> (w1574:bool)
        n874 = local read "复位"() -> (w1575:bool)
        n875 = local read "复位"() -> (w1577:bool)
        n876 = local read "红灯"() -> (w1576:bool)
        n877 = case shown="真" w1572 {
          frame False {
            "红灯" <- TRUE ("红灯")
          }
          frame True {
            n878 = local write "红灯"(FALSE ("红灯")) -> ()
          }
        }
        n879 = Or(x=w1574, y=w1575) -> (x .or. y?=w1573:bool)
        n880 = case shown="真" w1573 {
          frame False {
          }
          frame True {
            n881 = local write "回零完成"(FALSE ("夹头夹紧控制")) -> ()
          }
        }
        n882 = local read "停止"() -> (w1579:bool)
        n883 = Compound Arithmetic op=OR(w1577, w1579, w1576) -> (w1578:bool)
        n884 = case shown="真" w1578 {
          frame False {
          }
          frame True {
            n885 = local read "测头机构电机"() -> (w1583:u32)
            n886 = local read "旋转齿条电机"() -> (w1584:u32)
            n887 = local read "电动缸电机"() -> (w1585:u32)
            n888 = call "PCI1220U停止.vi"("AxisHandle IN"=w1584) -> ()  [unwired: 9 in, 2 out]
            n889 = call "PCI1220U停止.vi"("AxisHandle IN"=w1585) -> ()  [unwired: 9 in, 2 out]
            n890 = call "PCI1220U停止.vi"("AxisHandle IN"=w1583) -> ()  [unwired: 9 in, 2 out]
          }
        }
      }
      frame #5 {
        n891 = local read "齿条扭矩(Nm)"() -> (w1588:dbl)
        n892 = local read "黄灯"() -> (w1586:bool)
        n893 = local read "旋转齿条轴左转"() -> (w1594:bool)
        n894 = Absolute Value(x=w1588) -> (abs(x)=w1593:dbl)
        n895 = local read "旋转齿条轴右转"() -> (w1589:bool)
        n896 = Not(x=w1594) -> (.not. x?=w1590:bool)
        n897 = Less?(x=w1593, y=20.0) -> (x < y?=w1591:bool)
        n898 = Compound Arithmetic op=AND(w1589, w1590, w1591, w1586) -> (w1587:bool)
        n899 = case shown="真" w1587 {
          frame False {
          }
          frame True {
            n900 = flat-sequence {
              tunnel: [w1598] -> w1596
              tunnel: w1596 -> [w1600]
              tunnel: [w1600] -> w1595
              tunnel: w1595 -> [w1611]
              frame #0 {
                n901 = local read "旋转齿条电机"() -> (w1597:u32)
                n902 = call "PCI1220U运行.vi"("方向"=enum32{"Negative", "Positive"}."Negative" ("Direction"), "AxisHandle IN"=w1597) -> ("AxisHandle OUT"=w1598:u32)  [unwired: 9 in]
              }
              frame #1 {
                n903 = while {
                  stop <- w1604 stop-if-true
                  n904 = Wait (ms)(milliseconds to wait=u32 50 ("毫秒倍数")) -> ()  [unwired: 1 out]
                  n905 = local read "齿条扭矩(Nm)"() -> (w1609:dbl)
                  n906 = local read "旋转齿条轴右转"() -> (w1606:bool)
                  n907 = local read "红灯"() -> (w1601:bool)
                  n908 = local read "复位"() -> (w1602:bool)
                  n909 = Absolute Value(x=w1609) -> (abs(x)=w1608:dbl)
                  n910 = Not(x=w1606) -> (.not. x?=w1603:bool)
                  n911 = Greater?(x=w1608, y=10.0) -> (0:w1605:bool)
                  n912 = Compound Arithmetic op=OR(w1605, w1603, w1602, w1601) -> (w1604:bool)
                }
              }
              frame #2 {
                n913 = call "PCI1220U停止.vi"("AxisHandle IN"=w1611) -> ()  [unwired: 9 in, 2 out]
              }
            }
          }
        }
      }
      frame #6 {
        n914 = local read "齿条扭矩(Nm)"() -> (w1616:dbl)
        n915 = local read "旋转齿条轴右转"() -> (w1620:bool)
        n916 = Absolute Value(x=w1616) -> (abs(x)=w1615:dbl)
        n917 = local read "旋转齿条轴左转"() -> (w1618:bool)
        n918 = local read "黄灯"() -> (w1612:bool)
        n919 = Not(x=w1620) -> (.not. x?=w1617:bool)
        n920 = Less?(x=w1615, y=20.0) -> (x < y?=w1613:bool)
        n921 = Compound Arithmetic op=AND(w1618, w1617, w1613, w1612) -> (w1619:bool)
        n922 = case shown="真" w1619 {
          frame False {
          }
          frame True {
            n923 = flat-sequence {
              tunnel: [w1624] -> w1622
              tunnel: w1622 -> [w1626]
              tunnel: [w1626] -> w1621
              tunnel: w1621 -> [w1637]
              frame #0 {
                n924 = local read "旋转齿条电机"() -> (w1623:u32)
                n925 = call "PCI1220U运行.vi"("方向"=enum32{"Negative", "Positive"}."Positive" ("Direction"), "AxisHandle IN"=w1623) -> ("AxisHandle OUT"=w1624:u32)  [unwired: 9 in]
              }
              frame #1 {
                n926 = while {
                  stop <- w1629 stop-if-true
                  n927 = Wait (ms)(milliseconds to wait=u32 50 ("毫秒倍数")) -> ()  [unwired: 1 out]
                  n928 = local read "齿条扭矩(Nm)"() -> (w1635:dbl)
                  n929 = local read "旋转齿条轴左转"() -> (w1632:bool)
                  n930 = local read "红灯"() -> (w1627:bool)
                  n931 = local read "复位"() -> (w1628:bool)
                  n932 = Absolute Value(x=w1635) -> (abs(x)=w1634:dbl)
                  n933 = Not(x=w1632) -> (.not. x?=w1630:bool)
                  n934 = Greater?(x=w1634, y=10.0) -> (0:w1631:bool)
                  n935 = Compound Arithmetic op=OR(w1628, w1627, w1631, w1630) -> (w1629:bool)
                }
              }
              frame #2 {
                n936 = call "PCI1220U停止.vi"("AxisHandle IN"=w1637) -> ()  [unwired: 9 in, 2 out]
              }
            }
          }
        }
      }
      frame #7 {
        n937 = local read "齿条推拉力(N)"() -> (w1642:dbl)
        n938 = local read "电动缸前进"() -> (w1639:bool)
        n939 = local read "电动缸后退"() -> (w1638:bool)
        n940 = Absolute Value(x=w1642) -> (abs(x)=w1646:dbl)
        n941 = local read "黄灯"() -> (w1640:bool)
        n942 = Not(x=w1638) -> (.not. x?=w1643:bool)
        n943 = Less?(x=w1646, y=1000.0) -> (x < y?=w1644:bool)
        n944 = Compound Arithmetic op=AND(w1639, w1643, w1640, w1644) -> (w1641:bool)
        n945 = case shown="真" w1641 {
          frame False {
          }
          frame True {
            n946 = flat-sequence {
              tunnel: [w1650] -> w1648
              tunnel: w1648 -> [w1652]
              tunnel: [w1652] -> w1647
              tunnel: w1647 -> [w1663]
              frame #0 {
                n947 = local read "电动缸电机"() -> (w1649:u32)
                n948 = call "PCI1220U运行.vi"("方向"=enum32{"Negative", "Positive"}."Positive" ("Direction"), "AxisHandle IN"=w1649) -> ("AxisHandle OUT"=w1650:u32)  [unwired: 9 in]
              }
              frame #1 {
                n949 = while {
                  stop <- w1660 stop-if-true
                  n950 = local read "电动缸前进"() -> (w1657:bool)
                  n951 = local read "齿条推拉力(N)"() -> (w1654:dbl)
                  n952 = Wait (ms)(milliseconds to wait=u32 50 ("毫秒倍数")) -> ()  [unwired: 1 out]
                  n953 = Absolute Value(x=w1654) -> (abs(x)=w1656:dbl)
                  n954 = local read "红灯"() -> (w1658:bool)
                  n955 = local read "复位"() -> (w1659:bool)
                  n956 = Greater?(x=w1656, y=1000.0) -> (0:w1653:bool)
                  n957 = Not(x=w1657) -> (.not. x?=w1661:bool)
                  n958 = Compound Arithmetic op=OR(w1659, w1658, w1661, w1653) -> (w1660:bool)
                }
              }
              frame #2 {
                n959 = call "PCI1220U停止.vi"("AxisHandle IN"=w1663) -> ()  [unwired: 9 in, 2 out]
              }
            }
          }
        }
      }
      frame #8 {
        n960 = local read "电动缸前进"() -> (w1664:bool)
        n961 = local read "齿条推拉力(N)"() -> (w1668:dbl)
        n962 = local read "电动缸后退"() -> (w1665:bool)
        n963 = Absolute Value(x=w1668) -> (abs(x)=w1672:dbl)
        n964 = local read "黄灯"() -> (w1666:bool)
        n965 = Not(x=w1664) -> (.not. x?=w1669:bool)
        n966 = Less?(x=w1672, y=1000.0) -> (x < y?=w1670:bool)
        n967 = Compound Arithmetic op=AND(w1665, w1669, w1666, w1670) -> (w1667:bool)
        n968 = case shown="真" w1667 {
          frame False {
          }
          frame True {
            n969 = flat-sequence {
              tunnel: [w1676] -> w1674
              tunnel: w1674 -> [w1678]
              tunnel: [w1678] -> w1673
              tunnel: w1673 -> [w1689]
              frame #0 {
                n970 = local read "电动缸电机"() -> (w1675:u32)
                n971 = call "PCI1220U运行.vi"("方向"=enum32{"Negative", "Positive"}."Negative" ("Direction"), "AxisHandle IN"=w1675) -> ("AxisHandle OUT"=w1676:u32)  [unwired: 9 in]
              }
              frame #1 {
                n972 = while {
                  stop <- w1686 stop-if-true
                  n973 = local read "电动缸后退"() -> (w1683:bool)
                  n974 = local read "齿条推拉力(N)"() -> (w1682:dbl)
                  n975 = Wait (ms)(milliseconds to wait=u32 50 ("毫秒倍数")) -> ()  [unwired: 1 out]
                  n976 = Absolute Value(x=w1682) -> (abs(x)=w1680:dbl)
                  n977 = local read "红灯"() -> (w1685:bool)
                  n978 = local read "复位"() -> (w1684:bool)
                  n979 = Greater?(x=w1680, y=1000.0) -> (0:w1679:bool)
                  n980 = Not(x=w1683) -> (.not. x?=w1687:bool)
                  n981 = Compound Arithmetic op=OR(w1684, w1685, w1687, w1679) -> (w1686:bool)
                }
              }
              frame #2 {
                n982 = call "PCI1220U停止.vi"("AxisHandle IN"=w1689) -> ()  [unwired: 9 in, 2 out]
              }
            }
          }
        }
      }
      frame #9 {
        n983 = local read "测头机构轴后退"() -> (w1690:bool)
        n984 = local read "测头机构轴前进"() -> (w1691:bool)
        n985 = local read "黄灯"() -> (w1692:bool)
        n986 = Not(x=w1690) -> (.not. x?=w1694:bool)
        n987 = Compound Arithmetic op=AND(w1691, w1694, w1692) -> (w1693:bool)
        n988 = case shown="真" w1693 {
          frame False {
          }
          frame True {
            n989 = flat-sequence {
              tunnel: [w1698] -> w1696
              tunnel: w1696 -> [w1700]
              tunnel: [w1700] -> w1695
              tunnel: w1695 -> [w1707]
              frame #0 {
                n990 = local read "测头机构电机"() -> (w1697:u32)
                n991 = call "PCI1220U运行.vi"("方向"=enum32{"Negative", "Positive"}."Positive" ("Direction"), "AxisHandle IN"=w1697) -> ("AxisHandle OUT"=w1698:u32)  [unwired: 9 in]
              }
              frame #1 {
                n992 = while {
                  stop <- w1704 stop-if-true
                  n993 = local read "测头机构轴前进"() -> (w1701:bool)
                  n994 = Wait (ms)(milliseconds to wait=u32 50 ("毫秒倍数")) -> ()  [unwired: 1 out]
                  n995 = local read "红灯"() -> (w1702:bool)
                  n996 = local read "复位"() -> (w1703:bool)
                  n997 = Not(x=w1701) -> (.not. x?=w1705:bool)
                  n998 = Compound Arithmetic op=OR(w1703, w1702, w1705) -> (w1704:bool)
                }
              }
              frame #2 {
                n999 = call "PCI1220U停止.vi"("AxisHandle IN"=w1707) -> ()  [unwired: 9 in, 2 out]
              }
            }
          }
        }
      }
      frame #10 {
        n1000 = local read "测头机构轴前进"() -> (w1708:bool)
        n1001 = local read "测头机构轴后退"() -> (w1709:bool)
        n1002 = local read "黄灯"() -> (w1710:bool)
        n1003 = Not(x=w1708) -> (.not. x?=w1712:bool)
        n1004 = Compound Arithmetic op=AND(w1709, w1712, w1710) -> (w1711:bool)
        n1005 = case shown="真" w1711 {
          frame False {
          }
          frame True {
            n1006 = flat-sequence {
              tunnel: [w1716] -> w1714
              tunnel: w1714 -> [w1718]
              tunnel: [w1718] -> w1713
              tunnel: w1713 -> [w1725]
              frame #0 {
                n1007 = local read "测头机构电机"() -> (w1715:u32)
                n1008 = call "PCI1220U运行.vi"("方向"=enum32{"Negative", "Positive"}."Negative" ("Direction"), "AxisHandle IN"=w1715) -> ("AxisHandle OUT"=w1716:u32)  [unwired: 9 in]
              }
              frame #1 {
                n1009 = while {
                  stop <- w1722 stop-if-true
                  n1010 = local read "测头机构轴后退"() -> (w1719:bool)
                  n1011 = Wait (ms)(milliseconds to wait=u32 50 ("毫秒倍数")) -> ()  [unwired: 1 out]
                  n1012 = local read "红灯"() -> (w1721:bool)
                  n1013 = local read "复位"() -> (w1720:bool)
                  n1014 = Not(x=w1719) -> (.not. x?=w1723:bool)
                  n1015 = Compound Arithmetic op=OR(w1720, w1721, w1723) -> (w1722:bool)
                }
              }
              frame #2 {
                n1016 = call "PCI1220U停止.vi"("AxisHandle IN"=w1725) -> ()  [unwired: 9 in, 2 out]
              }
            }
          }
        }
      }
    }
    n1017 = Wait (ms)(milliseconds to wait=u32 50 ("毫秒倍数")) -> ()  [unwired: 1 out]
    n1018 = local read "停止"() -> (w1512:bool)
  }
  n1019 = flat-sequence {
    tunnel: [w1729] -> w2
    tunnel: [w1727] -> w1
    tunnel: w2 -> [w1739]
    tunnel: w1 -> [w1738]
    frame #0 {
      n1020 = First Call?() -> (First Call?: T/F=w1726:bool)
      n1021 = case shown="真" w1726 {
        frame False {
        }
        frame True {
          n1022 = while {
            i -> [w1733]
            stop <- w1734 stop-if-true
            w1737 = TRUE ("电动缸使能")
            n1023 = Wait Until Next ms Multiple(millisecond multiple=u32 50 ("毫秒倍数")) -> ()  [unwired: 1 out]
            n1024 = local write "回零完成"(FALSE ("回零完成")) -> ()
            n1025 = local write "测头机构轴使能"(w1737) -> ()
            n1026 = local write "旋转齿条轴使能"(w1737) -> ()
            n1027 = local write "电动缸使能"(w1737) -> ()
            n1028 = Greater Or Equal?(x=w1733, y=u32 30) -> (x >= y?=w1734:bool)
          }
        }
      }
      n1029 = call "ADO Connection Create.vi"() -> ("error out"=w1730:errorcluster, "ADODB._Connection Out"=w1731:refnum<k7>)  [unwired: 10 in]
      n1030 = call "ADO Connection Open.vi"("error in (no error)"=w1730, "ConnectionString"="Provider=Microsoft.Jet.OLEDB.4.0;Data Source=D:\\Q14070-Z060人机界面\\参数\\参数Z060.mdb;Persist Security Info=False;Jet OLEDB:Database Password=123;", "ADODB._Connection In"=w1731) -> ("error out"=w1727:errorcluster, "ADODB._Connection Out"=w1729:refnum<k7>)  [unwired: 7 in]
    }
    frame #1 {
      n1031 = while {
        tunnel: w1739 -> [w1741]
        tunnel: w1738 -> [w1740]
        stop <- w1745 stop-if-true
        n1032 = Wait (ms)(milliseconds to wait=u32 50 ("等待时间（毫秒）")) -> ()  [unwired: 1 out]
        n1033 = First Call?() -> (First Call?: T/F=w1744:bool)
        n1034 = Or(x=w1744, y="参数加载") -> (x .or. y?=w1743:bool)
        n1035 = case shown="真" w1743 {
          tunnel: w1741 -> [_ w1748]
          tunnel: w1740 -> [_ w1747]
          frame False {
          }
          frame True {
            n1036 = stacked-sequence {
              tunnel: w1748 -> [w1754 w1803 w1822]
              tunnel: w1747 -> [w1749 _ _]
              frame #0 {
                n1037 = call "SQL Execute.vi"("error in (no error)"=w1749, "Command Text"="SELECT * FROM 测试参数表", "ADODB._Connection In"=w1754) -> ("Data"=w1752:string[][])  [unwired: 5 in, 3 out]
                n1038 = Index Array(array=w1752, index (col)=0 ("索引 (行)")) -> (element=w1756:string[])  [unwired: 1 in]
                n1039 = Array Size(array=w1756) -> (size(s)=w1751:i32)
                "型号数量" <- w1751
                n1040 = while {
                  shift-right: [w1763] -> w1755
                  shift-left: i32[] [] -> [w1762]
                  tunnel: w1751 -> [w1760]
                  i -> [w1761]
                  stop <- w1759 stop-if-true
                  n1041 = Greater Or Equal?(x=w1761, y=w1760) -> (x >= y?=w1759:bool)
                  n1042 = Build Array (concatenate)(w1762, w1761) -> (w1763:i32[])
                }
                n1043 = Build Cluster Array "索引与捆绑簇数组"(w1756, w1755) -> (w1750:cluster{"String":string, i32}[])
                n1044 = property on="型号选择" class="Ring (严格)"("StringsAndValues[]"=w1750) -> ()  [unwired: 2 in, 2 out]
              }
              frame #1 {
                n1045 = property on="型号选择" class="Ring (严格)"() -> ("RingText.Text"=w1804:string)  [unwired: 2 in, 2 out]
                n1046 = call "创建文本2"("型号选择"=w1804) -> ("Result"=w1808:string)  [unwired: 13 in, 1 out]
                n1047 = call "SQL Execute.vi"("Command Text"=w1808, "ADODB._Connection In"=w1803) -> ("Data"=w1807:string[][])  [unwired: 6 in, 3 out]
                n1048 = Index Array(array=w1807, index (row)=0 ("索引 (行)")) -> (element=w1805:string[])  [unwired: 1 in]
                n1049 = Fract/Exp String To Number ("分数/指数字符串至数值转换")(string=w1805) -> (number=w1792:dbl[])  [unwired: 3 in, 1 out]
                n1050 = Index Array ("索引数组")(array=w1792, index #1=2 ("索引"), index #2=3 ("索引"), index #3=4 ("索引"), index #4=5 ("索引"), index #5=6 ("索引"), index #6=7 ("索引"), index #7=8 ("索引"), index #8=9 ("索引"), index #9=10 ("索引"), index #10=11 ("索引"), index #11=12 ("索引"), index #12=13 ("索引"), index #13=14 ("索引"), index #14=15 ("索引"), index #15=16 ("索引"), index #16=17 ("索引"), index #17=18 ("索引"), index #18=19 ("索引"), index #19=20 ("索引")) -> (element #1=w1791:dbl, element #2=w1790:dbl, element #3=w1789:dbl, element #4=w1788:dbl, element #5=w1787:dbl, element #6=w1786:dbl, element #7=w1785:dbl, element #8=w1784:dbl, element #9=w1783:dbl, element #10=w1782:dbl, element #11=w1781:dbl, element #12=w1780:dbl, element #13=w1774:dbl, element #14=w1773:dbl, element #15=w1772:dbl, element #16=w1771:dbl, element #17=w1767:dbl, element #18=w1766:dbl, element #19=w1764:dbl)
                n1051 = local write "测头机构轴移动速度"(w1791) -> ()
                n1052 = local write "测头机构轴检测位"(w1790) -> ()
                n1053 = local write "测头机构轴后退位"(w1788) -> ()
                n1054 = local write "测头机构轴待检位"(w1789) -> ()
                n1055 = local write "旋转伺服找帽转速"(w1784) -> ()
                n1056 = local write "旋转伺服测量转速"(w1783) -> ()
                n1057 = local write "总行程标准(mm)"(w1781) -> ()
                n1058 = local write "齿条移动速度"(w1787) -> ()
                n1059 = local write "平均轴向力MAX(N)"(w1771) -> ()
                n1060 = local write "最大轴向力标准(N)"(w1774) -> ()
                n1061 = local write "齿条左极限"(w1786) -> ()
                n1062 = local write "总行程最大值"(w1780) -> ()
                n1063 = local write "齿条右极限"(w1785) -> ()
                n1064 = local write "转向器中心"(w1764) -> ()
                n1065 = local write "总圈数标准"(w1767) -> ()
                n1066 = local write "总圈数最大值"(w1766) -> ()
                n1067 = local write "测量点扭矩"(w1782) -> ()
                n1068 = local write "力波动标准(N)"(w1773) -> ()
                n1069 = local write "轴向力标准(N)"(w1772) -> ()
              }
              frame #2 {
                n1070 = call "SQL Execute.vi"("Command Text"="SELECT * FROM 传感器校验表 where ID='1'", "ADODB._Connection In"=w1822) -> ("Data"=w1824:string[][])  [unwired: 6 in, 3 out]
                n1071 = Index Array(array=w1824) -> (element=w1825:string[])  [unwired: 2 in]
                n1072 = Fract/Exp String To Number ("分数/指数字符串至数值转换")(string=w1825) -> (number=w1815:dbl[])  [unwired: 3 in, 1 out]
                n1073 = Index Array(array=w1815, index #1=1 ("索引"), index #2=2 ("索引"), index #3=3 ("索引"), index #4=4 ("索引"), index #5=5 ("索引"), index #6=6 ("索引")) -> (element #1=w1814:dbl, element #2=w1813:dbl, element #3=w1812:dbl, element #4=w1811:dbl, element #5=w1810:dbl, element #6=w1809:dbl)
                n1074 = local write "间隙位移零点偏移"(w1814) -> ()
                n1075 = local write "间隙位移比例偏移"(w1813) -> ()
                n1076 = local write "齿条推拉力零点偏移"(w1812) -> ()
                n1077 = local write "齿条推拉力比例偏移"(w1811) -> ()
                n1078 = local write "齿条扭矩零点偏移"(w1810) -> ()
                n1079 = local write "齿条扭矩比例偏移"(w1809) -> ()
              }
            }
          }
        }
        n1080 = local read "停止"() -> (w1745:bool)
        "ADODB._Connection Out 2" <- w1741
      }
    }
  }
  n1081 = while {
    stop <- w1827 stop-if-true
    n1082 = local read "rfid工步号"() -> (w1826:u32)
    n1083 = case shown="10" w1826 {
      frame 0, Default {
      }
      frame 10 {
        n1084 = flat-sequence {
          tunnel: [w1837] -> w1831
          tunnel: w1831 -> [w1841]
          tunnel: [w1838] -> w1830
          tunnel: w1830 -> [w1843]
          tunnel: [w1843] -> w1829
          tunnel: w1829 -> [w1846]
          frame #0 {
            n1085 = while {
              stop <- w1832 stop-if-true
              n1086 = local read "rfid触发"() -> (w1832:bool)
              n1087 = Wait Until Next ms Multiple(millisecond multiple=u32 50 ("毫秒倍数")) -> ()  [unwired: 1 out]
            }
          }
          frame #1 {
            n1088 = local write "芯片ID"("" ("随行板ID")) -> ()
            n1089 = local write "rfid完成"(FALSE ("RFID完成")) -> ()
            n1090 = local write "rfid触发"(FALSE ("RFID读取触发")) -> ()
          }
          frame #2 {
            n1091 = local read "Z060ARFID"() -> (w1837:string)
            n1092 = local write "芯片ID"(w1837) -> ()
          }
          frame #3 {
            w1839 = T6 0 items=["两端", "字符串首端", "字符串末端"] ("location (both)")
            n1093 = call "查询产品ID.vi"("芯片编码"=w1841) -> ("产品ID"=w1840:string)  [unwired: 8 in, 2 out]
            "读取产品ID" <- w1840
            n1094 = call <vilib>:"Trim Whitespace.vi"("string"=w1840, "location (both)"=w1839) -> ("trimmed string"=w1838:string)
          }
          frame #4 {
            n1095 = Wait Until Next ms Multiple(millisecond multiple=u32 500 ("毫秒倍数")) -> ()  [unwired: 1 out]
          }
          frame #5 {
            n1096 = call "查询上序合格.vi"("产品ID"=w1846) -> ("本序已做"=w1844:bool, "上序合格"=w1845:bool)  [unwired: 8 in, 1 out]
            n1097 = Not(x=w1845) -> (.not. x?=w1847:bool)
            n1098 = local write "上序不合格"(w1847) -> ()
            n1099 = local write "上序合格"(w1845) -> ()
            n1100 = local write "本序已做"(w1844) -> ()
          }
          frame #6 {
            n1101 = local write "rfid完成"(TRUE ("RFID读取完成")) -> ()
            n1102 = Wait Until Next ms Multiple(millisecond multiple=u32 500 ("毫秒倍数")) -> ()  [unwired: 1 out]
          }
          frame #7 {
            "rfid工步号" <- 15.0 ("工步号")
          }
        }
      }
      frame 210 {
        n1103 = local read "读取产品ID"() -> (w1851:string)
        n1104 = local write "产品ID"(w1851) -> ()
      }
    }
    n1105 = Wait Until Next ms Multiple(millisecond multiple=u32 50 ("毫秒倍数")) -> ()  [unwired: 1 out]
    n1106 = local read "停止"() -> (w1827:bool)
  }
  n1107 = flat-sequence {
    tunnel: [w1852] -> w4
    tunnel: w4 -> [w1858]
    tunnel: [w1857] -> w3
    tunnel: w3 -> [w1928]
    frame #0 {
      n1108 = call "PCI1240U初始化.vi"() -> ("旋转电机"=→"旋转齿条电机":u32, "电动缸电机"=→"电动缸电机":u32, "DeviceHandle"=→"DeviceHandle":u32, "进给电机"=→"测头机构电机":u32)  [unwired: 6 in, 2 out]
      n1109 = call "PCI8622配置.vi"() -> ("DeviceID"=w1852:i32)  [unwired: 11 in]
    }
    frame #1 {
      n1110 = while {
        tunnel: w1858 -> [w1860]
        tunnel: [w1859] -> w1857
        stop <- "停止" stop-if-true
        n1111 = stacked-sequence {
          tunnel: w1860 -> [_ _ w1904]
          tunnel: [_ _ w1904] -> w1859
          frame #0 {
            n1112 = local read "测头机构电机"() -> (w1869:u32)
            n1113 = Boolean To (0,1)(Boolean="测头机构轴使能") -> (0, 1=w1867:i16)
            n1114 = call <userlib>:"Acm_AxSetSvOn.vi"("OnOff"=w1867, "AxisHandle"=w1869) -> ("AxisHandle"=w1866:u32)  [unwired: 1 in, 2 out]
            n1115 = call "PCI1220U进给轴速度设置.vi"("Change Velocity"="测头机构轴速度(mm/s)", "AxisHandle IN"=w1866) -> ("AxisHandle OUT"=w1864:u32)  [unwired: 9 in]
            n1116 = call "PCI1220U进给轴读取位置.vi"("AxisHandle IN"=w1864) -> ("位置"=→"测头机构轴位置(mm)":dbl)  [unwired: 9 in, 1 out]
          }
          frame #1 {
            n1117 = local read "电动缸电机"() -> (w1879:u32)
            n1118 = local read "旋转齿条电机"() -> (w1878:u32)
            n1119 = Boolean To (0,1)(Boolean="电动缸使能") -> (0, 1=w1883:i16)
            n1120 = Boolean To (0,1)(Boolean="旋转齿条轴使能") -> (0, 1=w1877:i16)
            n1121 = call <userlib>:"Acm_AxSetSvOn.vi"("OnOff"=w1877, "AxisHandle"=w1878) -> ("AxisHandle"=w1880:u32)  [unwired: 1 in, 2 out]
            n1122 = call <userlib>:"Acm_AxSetSvOn.vi"("OnOff"=w1883, "AxisHandle"=w1879) -> ("AxisHandle"=w1882:u32)  [unwired: 1 in, 2 out]
            n1123 = call "PCI1220U扭矩轴速度设置.vi"("Change Velocity"="旋转伺服速度(°/s)", "AxisHandle IN"=w1880) -> ("AxisHandle OUT"=w1881:u32)  [unwired: 9 in]
            n1124 = call "PCI1240电动缸速度设置.vi"("Change Velocity"="电动缸速度(mm/s)", "AxisHandle IN"=w1882) -> ("AxisHandle OUT"=w1870:u32)  [unwired: 9 in]
            n1125 = call "PCI1220U扭矩轴读取位置.vi"("AxisHandle IN"=w1881) -> ("位置"=→"旋转伺服位置(°)":dbl)  [unwired: 9 in, 1 out]
            n1126 = call "PCI1240电动缸读取位置.vi"("AxisHandle IN"=w1870) -> ("位置"=→"电动缸位置(mm)":dbl)  [unwired: 9 in, 1 out]
          }
          frame #2 {
            w1920 = 0  # nRetSizeWords
            w1921 = 2048  # nReadSizeWords
            # "hDevice"
            n1127 = Initialize Array(u16 0, 2048 ("dimension size")) -> (w1911:u16[])
            n1128 = dll-call lib="PCI8622_32.dll" fn="PCI8622_ReadDeviceProAD_Npt" label="ReadDeviceProAD_Npt"("hDevice"=w1904, "ADBuffer[]"=w1911, "nReadSizeWords"=w1921, "nRetSizeWords"=w1920) -> ("ADBuffer[]"=w1914:u16[])  [unwired: 7 in, 2 out]
            n1129 = Divide(x=w1914, y=65536.01) -> (x/y=w1915:dbl[])
            n1130 = Multiply(x=w1915, y=20) -> (x*y=w1918:dbl[])
            n1131 = Subtract(x=w1918, y=10) -> (x-y=w1910:dbl[])
            n1132 = Decimate 1D Array ("抽取一维数组")(w1910) -> (w1898:dbl[], w1899:dbl[], w1897:dbl[])  [unwired: 5 out]
            n1133 = Add Array Elements(numeric array=w1898) -> (sum=w1907:dbl)
            n1134 = Add Array Elements(numeric array=w1897) -> (sum=w1908:dbl)
            n1135 = Array Size(array=w1898) -> (size(s)=w1906:i32)
            n1136 = Add Array Elements(numeric array=w1899) -> (sum=w1903:dbl)
            n1137 = Array Size(array=w1897) -> (size(s)=w1909:i32)
            n1138 = Array Size(array=w1899) -> (size(s)=w1905:i32)
            n1139 = Divide(x=w1907, y=w1906) -> (x/y=w1896:dbl)
            n1140 = Divide(x=w1908, y=w1909) -> (x/y=w1888:dbl)
            n1141 = Divide(x=w1903, y=w1905) -> (x/y=w1893:dbl)
            n1142 = Subtract(x=w1888, y=2.371) -> (x-y=w1886:dbl)
            n1143 = Multiply(x=w1896, y=2.0) -> (x*y=w1891:dbl)
            n1144 = Multiply(x=w1893, y=200.0) -> (x*y=w1892:dbl)
            n1145 = Subtract(x=w1891, y=-1.0) -> (x-y=w1889:dbl)
            n1146 = Multiply(x=w1886, y=0.75) -> (x*y=w1884:dbl)
            n1147 = local read "间隙位移比例偏移"() -> (w1925:dbl)
            n1148 = local read "间隙位移零点偏移"() -> (w1924:dbl)
            n1149 = local read "齿条扭矩零点偏移"() -> (w1926:dbl)
            n1150 = local read "齿条扭矩比例偏移"() -> (w1927:dbl)
            n1151 = local read "齿条推拉力比例偏移"() -> (w1923:dbl)
            n1152 = local read "齿条推拉力零点偏移"() -> (w1922:dbl)
            n1153 = call "传感器校订.vi"("零点"=w1926, "比例"=w1927, "传感器"=w1889) -> ("示值"=→"齿条扭矩(Nm)":dbl)  [unwired: 8 in]
            n1154 = call "传感器校订.vi"("零点"=w1924, "比例"=w1925, "传感器"=w1884) -> ("示值"=→"间隙位移(mm)":dbl)  [unwired: 8 in]
            n1155 = call "传感器校订.vi"("零点"=w1922, "比例"=w1923, "传感器"=w1892) -> ("示值"=→"齿条推拉力(N)":dbl)  [unwired: 8 in]
          }
        }
        n1156 = Wait Until Next ms Multiple(millisecond multiple=u32 50 ("毫秒倍数")) -> ()  [unwired: 1 out]
      }
    }
    frame #2 {
      n1157 = dll-call lib="PCI8622_32.dll" fn="PCI8622_StopDeviceProAD" label="StopDeviceProAD"("hDevice"=w1928) -> ("hDevice"=w1929:i32)  [unwired: 4 in, 2 out]
      n1158 = dll-call lib="PCI8622_32.dll" fn="PCI8622_ReleaseDeviceProAD" label="ReleaseDeviceProAD"("hDevice"=w1929) -> ()  [unwired: 5 in, 2 out]
      n1159 = dll-call lib="PCI8622_32.dll" fn="PCI8622_ReleaseDevice" label="ReleaseDevice"("hDevice"=w1928) -> ()  [unwired: 5 in, 2 out]
    }
  }
